vi "MainCamera.vi"() -> ()   [LabVIEW 2018]
uses:
  VisionLibrariesXimea/xiLib/xiLIB_64bit/xiLIB/xiCamLib/xiLIB/Typedefs/xiLIB - PRM_Type.ctl
  VisionLibrariesXimea/xiLib/xiLIB_64bit/xiLIB/xiCamLib/xiLIB/Typedefs/xiLIB - PRM_Function.ctl
  VisionLibrariesXimea/xiLib/xiLIB_64bit/xiLIB/xiCamLib/xiCam/PRM/IMG_FORMAT/IMG_DATA_FORMAT.ctl
  VisionLibrariesXimea/xiLib/xiLIB_64bit/xiLIB/xiCamLib/xiCam/PRM/PRM/PRM_v2.ctl
  <vilib>/Utility/miscctls.llb/LVPointDoubleTypeDef.ctl
  typedef/StateMachineControl.ctl
  NetworkStream/NetworkStreamReceiverState.ctl
  typedef/StateProcessingLoop.ctl
  typedef/ImageUnit.ctl
  VisionLibrariesXimea/xiLib/xiLIB_64bit/xiLIB/xiCamLib/xiCam/PRM/BUFF_POLICY/BUFF_POLICY.ctl
  typedef/AcquisitionFrame.ctl
  NetworkStream/NetworkStreamData.ctl
  VisionLibrariesXimea/xiLib/xiLIB_64bit/xiLIB/xiCamLib/xiCam/PRM/ACQ_TIMING_MODE/ACQ_TIMING_MODE.ctl
  C:/XIMEA/API/x64/xiApi.NETX64.dll
  References.vi
  VisionLibrariesXimea/xiLib/xiLIB_64bit/xiLIB/xiCamLib/xiLIB/xiLIB - GetPRM_INFO.vi
  VisionLibrariesXimea/xiLib/xiLIB_64bit/xiLIB/xiCamLib/xiCam/Methods/xiCam - GetParam_Float.vi
  VisionLibrariesXimea/xiLib/xiLIB_64bit/xiLIB/xiCamLib/xiCam/Methods/xiCam - GetParam_String.vi
  Read and Save Files/FileType.ctl
  General Libraries/myFFT.lvlib
  Read and Save Files/RW_Protocols.lvlib
  General Libraries/Photon Filtering.lvlib
  General Libraries/statistics.lvlib
  NetworkStream/NetworkStream.lvlib
  <vilib>/dex/Stream Element Allocation Mode.ctl
  NetworkStream/NetworkStreamStateMachineVariable.ctl
  Shared program Control/MasterStatus.ctl
  Shared program Control/MySharedVariables.lvlib
panel:
  out "command error":errorcluster
  out "error out":errorcluster
  in  "?":T1(tab)
  in  "Stop Button":bool
  in  "Play Button":bool
  out "current sequence count":i32=10 min=1
  in  "Total sframe":i32=10 min=1
  in  "play sequence":bool
  in  "running mode":T2=enum."free run"
  out "status analysis":T2
  in  "buffer frames":i64=300
  out "# elements queue":i32
  in  "data analysis on":bool=TRUE
  out "efficiency to Main":dbl
  in  "data packing":bool
  in  "recent frame":bool
  in  "software Trigger":bool
  in  "Trigger ON":bool
  in  "Exposure (us)":i32(slide)=10 caption="Exposure (us) 1us - 1s steps of 1us" min=1 max=1000000 scale=0.9..5000.0
  in  "Gain":i32(slide) scale=0.0..10.0
  in  "IMG_FORMAT":T3
  in  "FrameRate":dbl(slide)=100.0 min=0.1 max=400.0 scale=0.0..400.0
  in  "TIMING MODE":i32
  in  "BUFF_POLICY":T4
  in  "auto-save ?":bool
  in  "name":string="Nbz0Nbx1_"
  in  "input PRM":T5=enum."IMAGE_DATA_FORMAT_RGB32_ALPHA"
  out "Type":T6
  out "Method":T7
  out "output":variant
  in  "is value??":bool
  in  "?":T8(tab)
  in  "Width Y":i32=1024 min=32 max=3424 step=32
  in  "Y-offset":i16=1312 min=0 max=3422 step=32
  in  "update ROI":bool
  out "ROI only":bool
  out "max RAM size (frame)":dbl
  in  "infos":bool
  in  "Save As Button":bool
  out "no frame dropping":bool
  out "Intensity Graph":u16[][](graph)
  in  "subwindow control":T10={"2^n : x"=10, "2^n : y"=10, "lower left box Position"={"X"=0.0, "Y"=0.0}, "Height (def 3424)"=0, "Width (def 4704)"=0} {"Width (def 4704)" min=32 max=3264; "Height (def 3424)" min=2 max=2634; "2^n : y" min=1 max=13; "2^n : x" min=1 max=13}
  out "time for acquire":dbl[unit] format="%#_2p"
  out "Enum":T11
  out "Network Stream State Indicator":T12
  out "skipped frames infos":T13
  out "loop":dbl[unit]
  out "required (Bytes) for single image":i32
  out "RAM size (frame)":dbl
  in  "Width X":i32=1024 min=32 max=4704 step=32
  in  "X-offset":i32=1760 min=0 max=2048 step=32
  out "buffer queue size":i32
  out "unit":string
  in  "minus BG":bool
  out "Ptot":dbl format="%#_4p"
  out "% saturation":dbl
  out "FFT":dbl[][](graph)
  in  "FFT int/phase":bool=TRUE
  in  "Filter on/off":bool=TRUE
  in  "filtered int/phase":bool=TRUE
  in  "Mask ON":bool
  out "filtered  FFT":dbl[][](graph)
  in  "unit":T14
  in  "Pause log":bool
  in  "info for log saving":string
  in  "clear graph":bool
  out "Waveform Chart":dbl(graph)
  out "timestamp":dbl
  out "shot noise std":dbl
  out "n":i32=10 min=1
  out "std":dbl
  out "mu":dbl
  out "STD":dbl[][](graph)
  out "MU":dbl[][](graph)
  in  "start stats":bool
  in  "Naverage 2D":i32=10
  in  "save name":string="phase"
  in  "start network scan":bool
  out "std scan":dbl
  out "mean scan":dbl
  out "network scan":dbl(graph)
  out "Sequence Number":u64
  in  "view snaps":bool
  in  "default BG":bool
  in  "Tab Control":T15(tab)
  out "BG":dbl[][](graph)
  in  "Snap":bool
  in  "Snap 2":bool
  out "REF":dbl[][](graph)
  in  "Snap 3":bool
  out "MAIN":dbl[][](graph)
  in  "Snap 4":bool
  out "REF+MAIN":dbl[][](graph)
  in  "phi(2) X":dbl
  in  "phi(2) Z":dbl
  in  "phi(1) X":dbl
  in  "phi(1) Z":dbl
  in  "Target Folder 2":path
  out "reconstructed image":dbl[][](graph)
  out "FFT acquire Graph":dbl[][](graph)
  in  "sequence list":i32[](listbox)
  in  "update loop":bool
  in  "N average":i32=3 min=1
  out "time for acquire":dbl[unit]
  out "timeout":bool=TRUE
  in  "Save result":bool
  in  "name 2":string="myResult"
  out "fft cluster":T16
  in  "sequence NbX NbZ":dbl[][](array[numeric])
  in  "fft cluster acquisition":T16
  in  "result array":dbl[][](array[numeric])
  out "sequence cluster":T17
  out "Array":i32[](array[numeric])
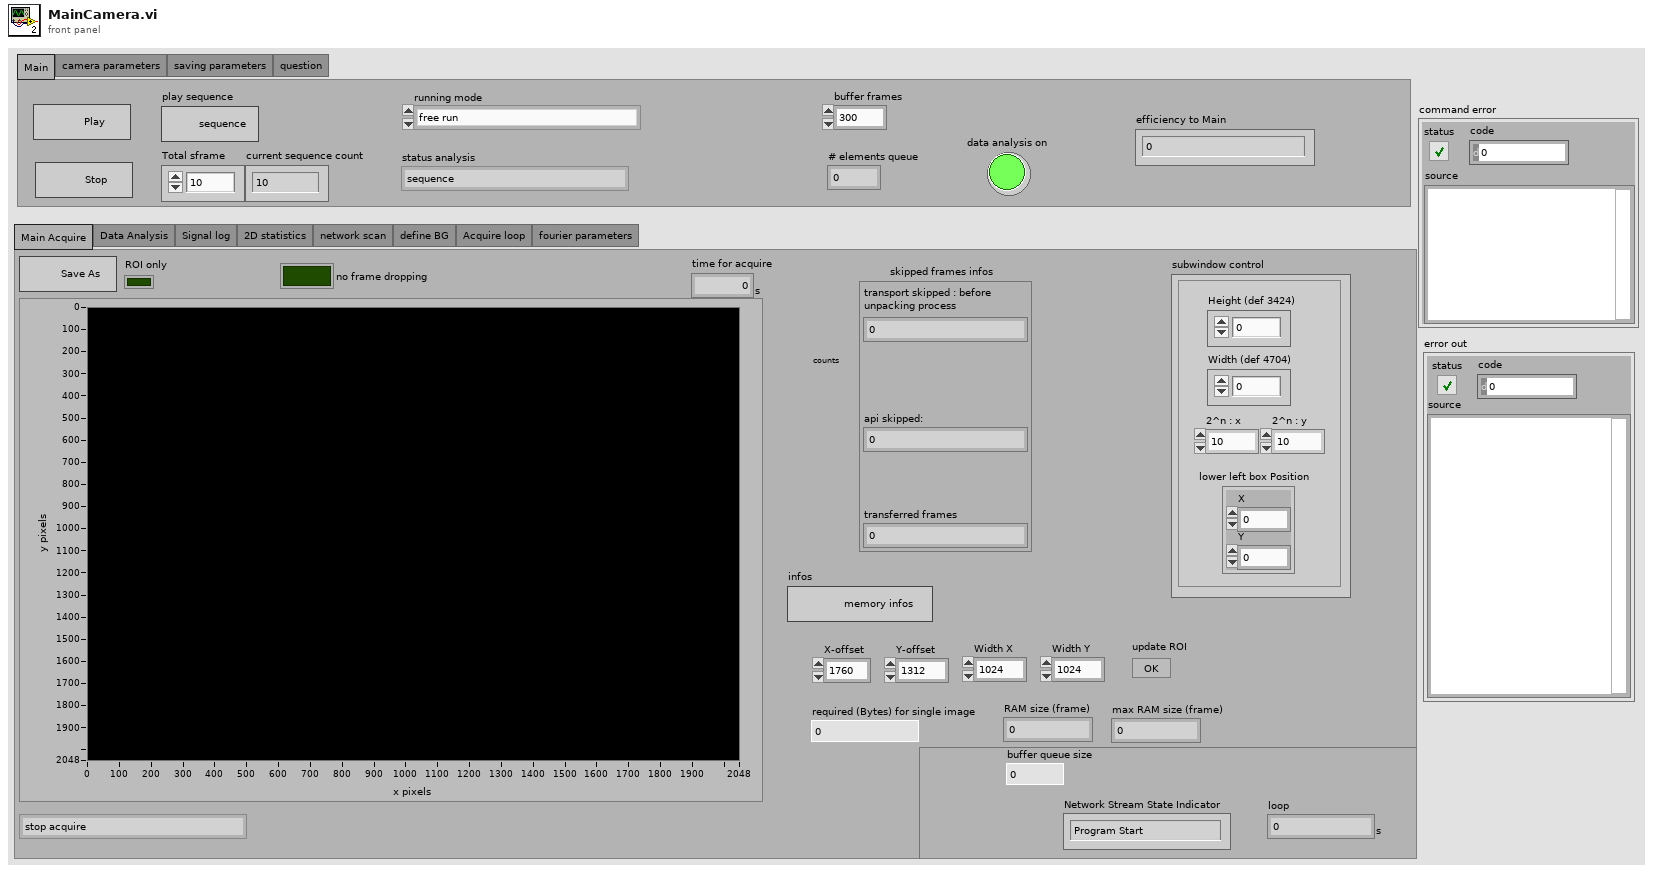
[diagram p1: front panel]
types:
  T1 = enum32{"Main", "camera parameters", "saving parameters", "question"}
  T2 = typedef "StateProcessingLoop.ctl" = enum16{"sequence", "Snap REF+MAIN", "Snap MAIN", "Snap REF", "Snap BG", "network sequence", "free run", "statistics"}
  T3 = typedef "IMG_DATA_FORMAT.ctl" = enum16{"MONO8", "MONO16", "RGB24", "RGB32", "RGBPLANAR", "RAW8", "RAW16"}
  T4 = typedef "BUFF_POLICY.ctl" = enum16{"UNSAFE", "SAFE"}
  T5 = typedef "PRM_v2.ctl" = enum16{"ACQ_BUFFER_SIZE", "ACQ_FRAME_BURST_COUNT", "ACQ_TIMING_MODE", "ACQ_TRANSPORT_BUFFER_SIZE", "AE_MAX_LIMIT", "AEAG", "AEAG_LEVEL", "API_VERSION", "AG_MAX_LIMIT", "APPLY_CMS", "AUTO_BANDWIDTH_CALCULATION", "AUTO_WB", "AVAILABLE_BANDWIDTH", "AVAILABLE_BANDWIDTH_MAX", "AVAILABLE_BANDWIDTH_MIN", "BPC", "BUFFER_POLICY", "BUFFERS_QUEUE_SIZE", "CC_MATRIX_00", "CC_MATRIX_01", "CC_MATRIX_02", "CC_MATRIX_03", "CC_MATRIX_10", "CC_MATRIX_11", "CC_MATRIX_12", "CC_MATRIX_13", "CC_MATRIX_20", "CC_MATRIX_21", "CC_MATRIX_22", "CC_MATRIX_23", "CC_MATRIX_30", "CC_MATRIX_31", "CC_MATRIX_32", "CC_MATRIX_33", "CHIP_TEMP", "CMS", "COLOR_FILTER_ARRAY", "COOLING", "DEBOUNCE_EN", "DEBOUNCE_POL", "DEBOUNCE_T0", "DEBOUNCE_T1", "DEBUG_LEVEL", "DEFAULT_CC_MATRIX", "DEVICE_INSTANCE_PATH", "DEVICE_MODEL_ID", "DEVICE_NAME", "DEVICE_SN", "DEVICE_TYPE", "DEVICE_USER_ID", "DOWNSAMPLING", "DOWNSAMPLING_MAX", "DOWNSAMPLING_MIN", "DOWNSAMPLING_TYPE", "DRV_VERSION", "EXP_PRIORITY", "EXPOSURE", "EXPOSURE_DIRECT_UPDATE", "EXPOSURE_MAX", "EXPOSURE_MIN", "FFS_FILE_NAME", "FPGA1_VERSION", "FRAMERATE", "FRAMERATE_MAX", "FRAMERATE_MIN", "FREE_FFS_SIZE", "GAIN", "GAIN_DIRECT_UPDATE", "GAIN_MAX", "GAIN_MIN", "GAMMAC", "GAMMAY", "GPI_LEVEL", "GPI_MODE", "GPI_SELECTOR", "GPI_SELECTOR_MAX", "GPI_SELECTOR_MIN", "GPO_MODE", "GPO_SELECTOR", "GPO_SELECTOR_MAX", "GPO_SELECTOR_MIN", "HDR", "HDR_T1", "HDR_T2", "HEIGHT", "HEIGHT_MAX", "HEIGHT_MIN", "HOUSE_TEMP", "IMAGE_DATA_FORMAT", "IMAGE_IS_COLOR", "INPUT_CMS_PROFILE", "IS_COOLED", "IS_DEVICE_EXIST", "KNEEPOINT1", "KNEEPOINT2", "LED_MODE", "LED_SELECTOR", "LED_SELECTOR_MAX", "LED_SELECTOR_MIN", "LIMIT_BANDWIDTH", "LIMIT_BANDWIDTH_MAX", "LIMIT_BANDWIDTH_MIN", "LUT_EN", "LUT_INDEX", "LUT_INDEX_MAX", "LUT_INDEX_MIN", "LUT_VALUE", "LUT_VALUE_MAX", "LUT_VALUE_MIN", "MANUAL_WB", "MCU1_VERSION", "MCU2_VERSION", "OFFSET_X", "OFFSET_X_MAX", "OFFSET_X_MIN", "OFFSET_Y", "OFFSET_Y_MAX", "OFFSET_Y_MIN", "OUTPUT_CMS_PROFILE", "OUTPUT_DATA_BIT_DEPTH", "OUTPUT_DATA_PACKING", "READ_FILE_FFS", "RECENT_FRAME", "SENSOR_DATA_BIT_DEPTH", "SENSOR_MODE", "SENSOR_TAPS", "SHARPNESS", "SHUTTER_TYPE", "TARGET_TEMP", "TRG_DELAY", "TRG_SELECTOR", "TRG_SOFTWARE", "TRG_SOURCE", "USED_FFS_SIZE", "WB_KB", "WB_KG", "WB_KR", "WIDTH", "WIDTH_MAX", "WIDTH_MIN", "WRITE_FILE_FFS", "ACQ_BUFFER_SIZE_UNIT", "ACQ_TRANSPORT_BUFFER_COMMIT", "AEAG_ROI_HEIGHT", "AEAG_ROI_OFFSET_X", "AEAG_ROU_OFFSET_Y", "AEAG_ROI_WIDTH", "API_CONTEXT_LIST", "BINNING_HORIZONTAL", "BINNING_SELECTOR", "BINNING_VERTICAL", "COLUMN_FPN_CORRECTION", "COUNTER_SELECTOR", "COUNTER_VALUE", "DECIMATION_HORIZONTAL", "DECIMATION_SELECTOR", "DECIMATION_VERTICAL", "DEVICE_ID", "DEVICE_LOCATION_PATH", "DEVICE_MANIFEST", "DEVICE_RESET", "DEVICE_SENS_SN", "EXPOSURE_BURST_COUNT", "FFS_ACCESS_KEY", "GAIN_SELECTOR", "HW_REVISION", "IMAGE_BLACK_LEVEL", "IMAGE_DATA_BIT_DEPTH", "IMAGE_DATA_FORMAT_RGB32_ALPHA", "IMAGE_PAYLOAD_SIZE", "LENS_APERTURE_VALUE", "LENS_FEATURE", "LENS_FEATURE_SELECTOR", "LENS_FOCAL_LENGTH", "LENS_FOCUS_DISTANCE", "LENS_FOCUS_MOVE", "LENS_FOCUS_MOVEMENT_VALUE", "LENS_MODE", "OUTPUT_DATA_PACKING_TYPE", "SENSOR_CLOCK_FREQ_HZ", "SENSOR_CLOCK_FREQ_INDEX", "SENSOR_FEATURE_SELECTOR", "SENSOR_FEATURE_VALUE", "SENSOR_OUTPUT_CHANNEL_COUNT", "TRANSPORT_PIXEL_FORMAT", "TS_RST_MODE", "TS_RST_SOURCE"}
  T6 = typedef "xiLIB - PRM_Type.ctl" = enum16{"Int32", "Float", "String", "DOWNSAMPLING_TYPE", "IMAGE_DATA_FORMAT", "BUFFER_POLICY", "TRG_SOURCE", "GPI", "GPO", "ACQ_TIMING_MODE", "BINNING_PATTERN", "BINNING_SELECTOR", "CMS_MODE", "COUNTER_SELECTOR", "DEBUG_LEVEL", "DECIMATION_PATTERN", "DECIMATION_SELECTOR", "GAIN_SELECTOR_TYPE", "LED_MODE", "LENS_FEATURE_SELECTOR", "LENS_MODE", "OUTPUT_DATA_PACKING_TYPE", "SENSOR_FEATURE_SELECTOR", "SHUTTER_TYPE", "TRG_SELECTOR", "TS_RST_MODE", "TS_RST_SOURCE"}
  T7 = typedef "xiLIB - PRM_Function.ctl" = enum16{"Get / Set", "Get", "Set"}
  T8 = enum32{"Main Acquire", "Data Analysis", "Signal log", "2D statistics", "network scan", "define BG", "Acquire loop", "fourier parameters"}
  T9 = typedef "LVPointDoubleTypeDef.ctl" = cluster{"X":dbl, "Y":dbl}
  T10 = cluster{"2^n : x":i8, "2^n : y":i8, "lower left box Position":T9, "Height (def 3424)":i32, "Width (def 4704)":i32}
  T11 = typedef "StateMachineControl.ctl" = enum16{"stop acquire", "acquire sequence", "wait", "start acquire sequence", "start acquire", "acquire"}
  T12 = typedef "NetworkStream.lvlib/NetworkStreamReceiverState.ctl" = enum16{"Program Start", "Waiting for connection", "Connected", "Connection lost", "Exit", "Unhandled Exception"}
  T13 = cluster{"transport skipped : before \nunpacking process ":i32, "api skipped: ":i32, "transferred frames":i32}
  T14 = typedef "ImageUnit.ctl" = enum16{"Nphotons", "Efficiency", "I(uW/cm^2)", "I(nW/cm^2)", "Nelectrons", "I[W/cm^2]", "counts"}
  T15 = enum32{"No field", "Ref only", "Main only", "Main + Ref no US"}
  T16 = cluster{"dFx":dbl, "dFy":dbl, "Nx":i32, "Ny":i32, "FxMax":dbl, "FyMax":dbl, "Xwidth":dbl, "Ywidth":dbl, "dx":dbl, "dy":dbl, "Fx points":dbl[], "X points":dbl[], "Y points":dbl[], "Fy points":dbl[]}
  T17 = cluster{"TypeOfSequence":string, "FreqSonde":dbl, "NbHemicycle":dbl, "Tau_cam":dbl, "DurWaveform":dbl, "Prof":dbl, "Nevent":i32, "nuX0":dbl, "nuZ0":dbl}
  T18 = typedef "NetworkStream.lvlib/NetworkStreamData.ctl" = cluster{"Command/Status":string, "Data":variant, "Session Hash":u64, "Sequence Number":u64}
  T19 = typedef "AcquisitionFrame.ctl" = cluster{"data array":u8[], "nframe":i32, "sframe":i32, "nframe0":i32, "data format":i32, "is sequence running ?":bool, "timestamp":dbl}
  T20 = typedef "ACQ_TIMING_MODE.ctl" = enum16{"FREE_RUN", "FRAME_RATE"}
  T21 = typedef "NetworkStream.lvlib/NetworkStreamStateMachineVariable.ctl" = cluster{"Network Stream Reader Endpoint":refnum<k21>, "Last Received Sequence Number":u64}
  T22 = typedef "Stream Element Allocation Mode.ctl" = u32
  T23 = cluster{"MU(1)":dbl[][], "MU(2)":dbl[][], "Ptot(1)":dbl, "Ptot(2)":dbl, "n":i32}
  T24 = cluster{"transport skipped":i32, "api skipped":i32, "transfert skipped":i32}
  T25 = typedef "MySharedVariables.lvlib/MasterStatus.ctl" = cluster{"Camera done":bool, "Tektronik done":bool, "Motors done":bool, "Gage done":bool}[]
  T26 = typedef "RW_Protocols.lvlib/FileType.ctl" = enum16{"png", "csv", "tiff", "dat", "bin", "txt"}
  T27 = cluster{"Filter on/off":bool, "filtered int/phase":bool, "Mask ON":bool, "FFT int/phase":bool}
  T28 = typedef "Photon Filtering.lvlib/OutputPhotonCluster.ctl" = cluster{"Unfiltered":dbl[][], "Ifft":dbl[][], "Ptot":dbl, "Tagged Photons":dbl[][], "% saturation":dbl, "efficiency":dbl, "variance coeff":dbl}
  T29 = cluster{"Camera done":bool, "Tektronik done":bool, "Motors done":bool, "Gage done":bool}
  T30 = cluster{"phi(1) X":dbl, "phi(1) Z":dbl, "phi(2) X":dbl, "phi(2) Z":dbl}
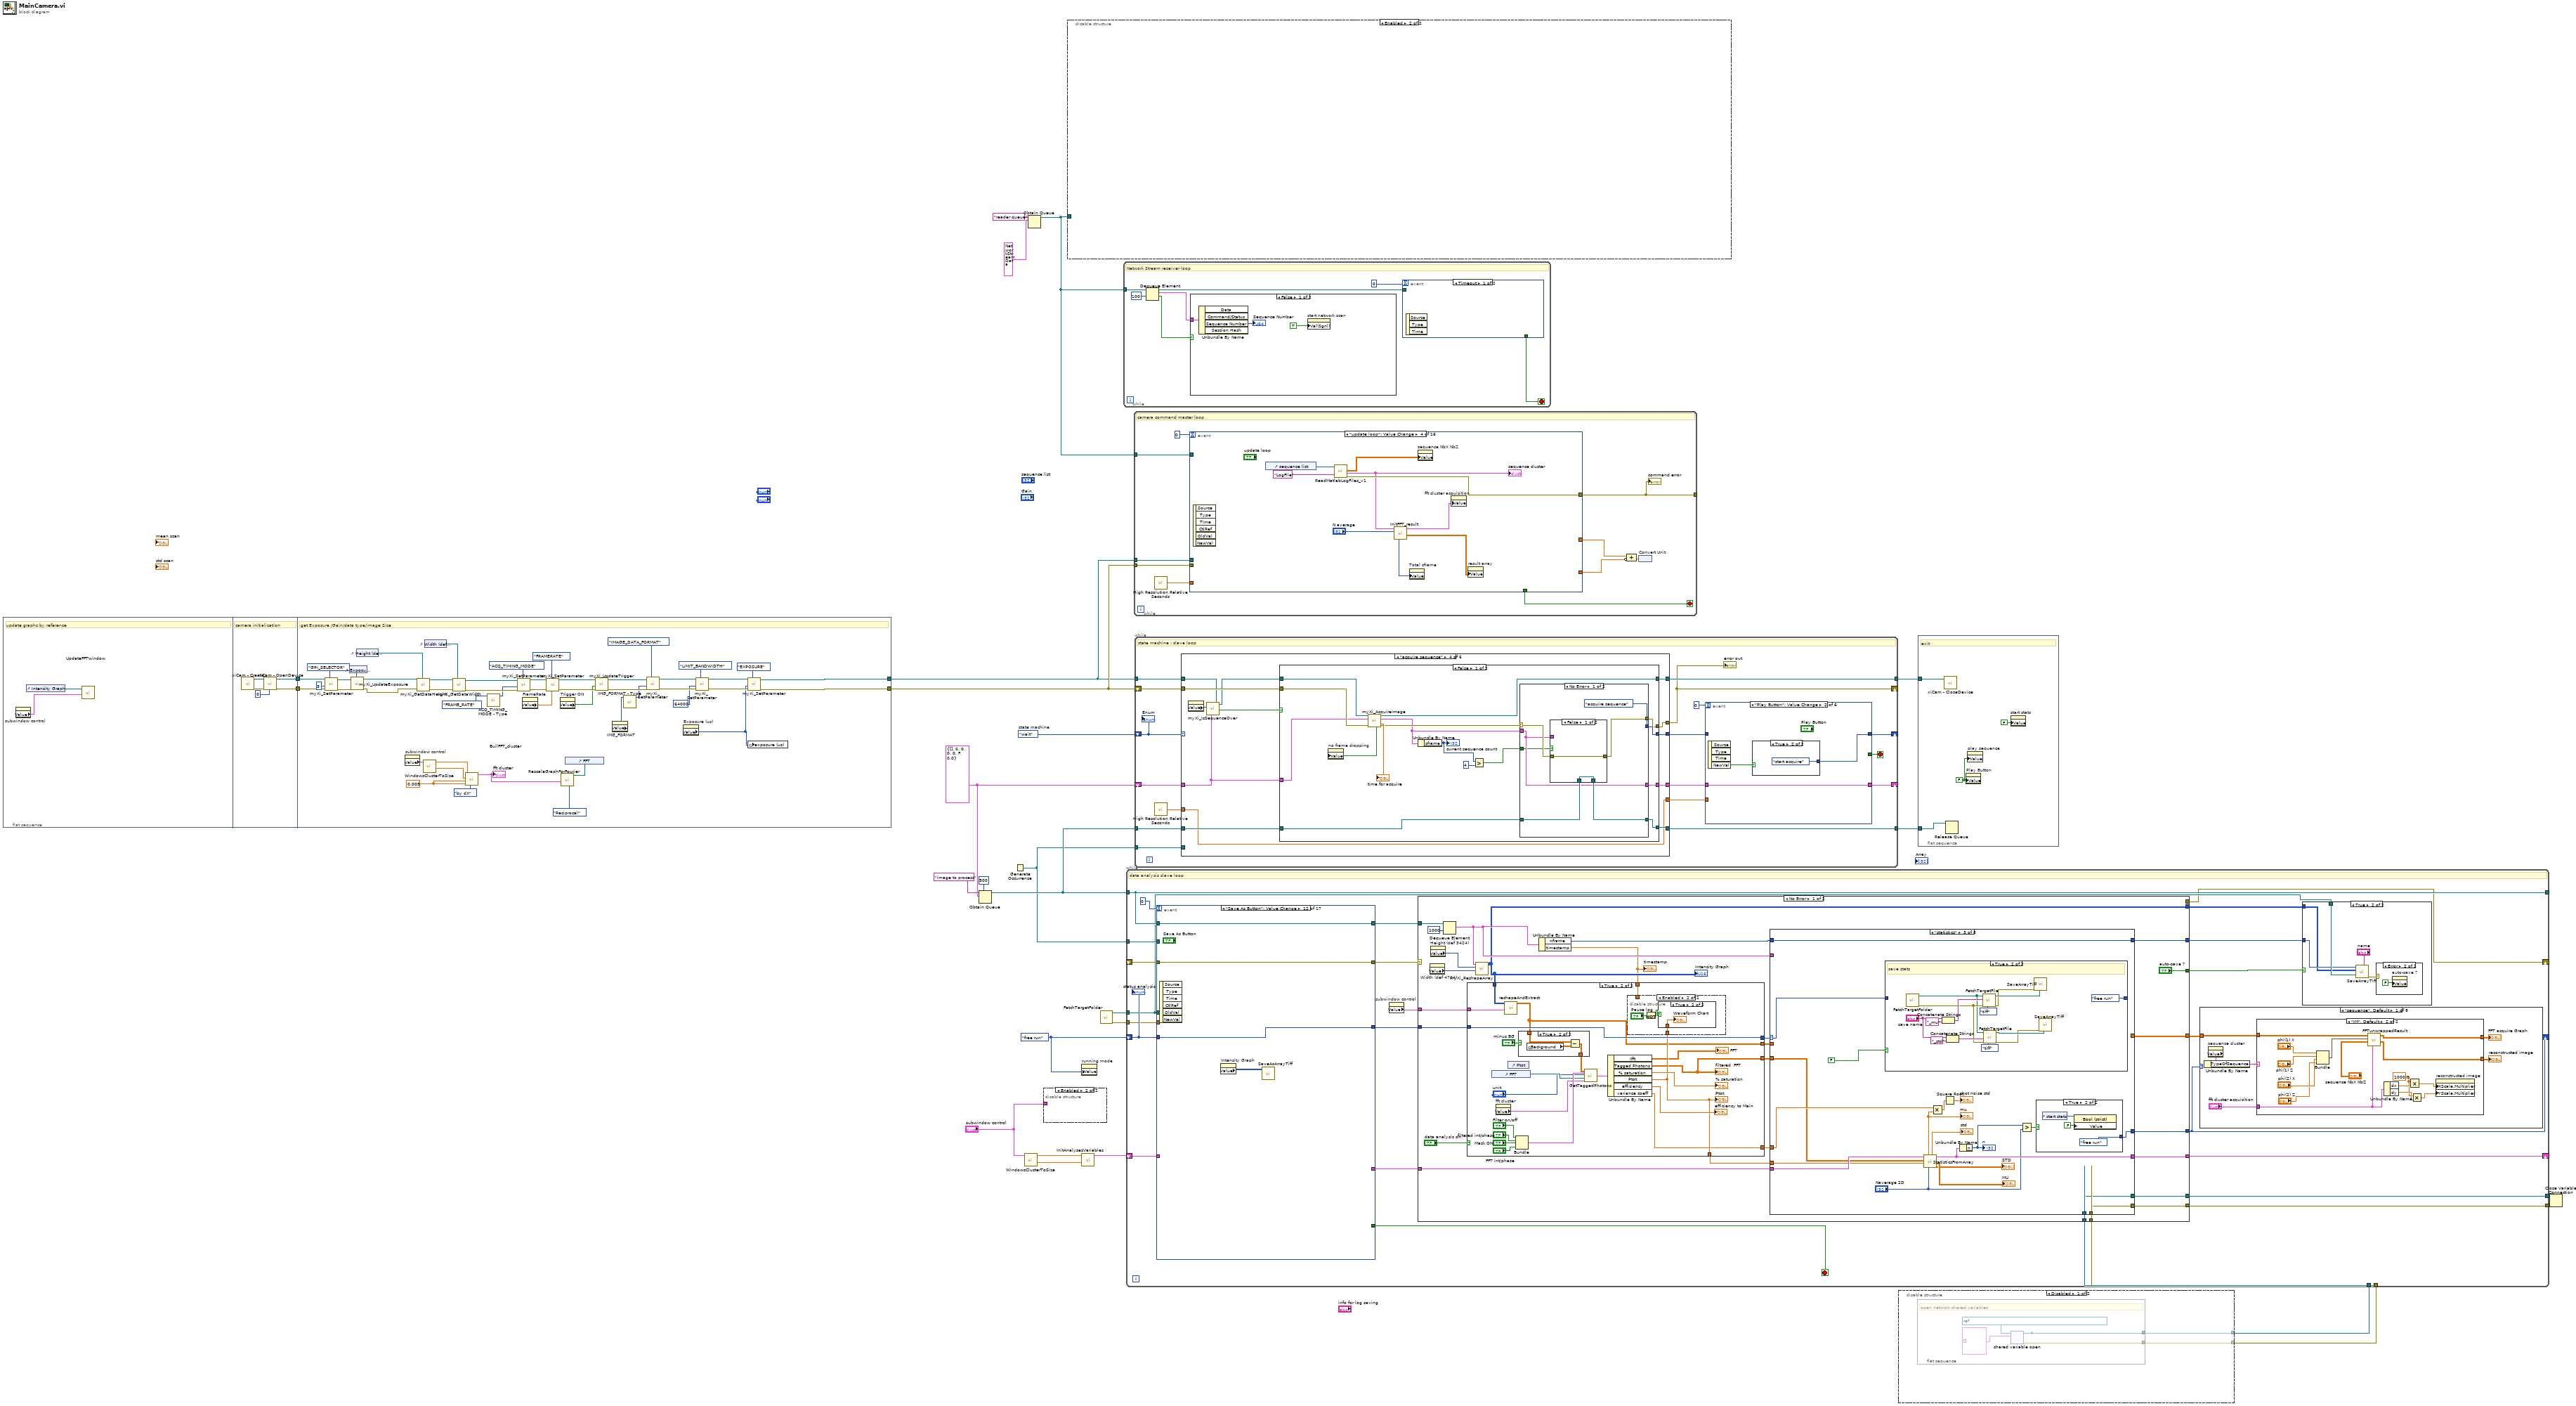
[diagram p0: block diagram]
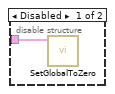
[diagram p2: hidden frame]
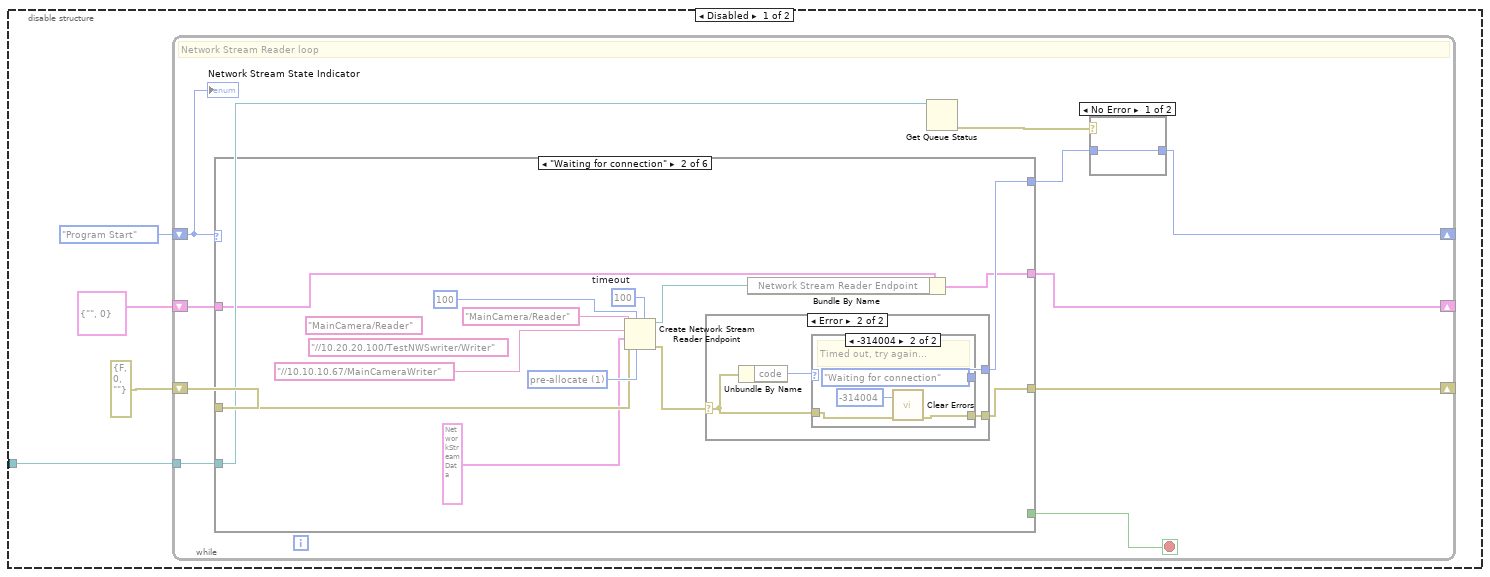
[diagram p4: hidden frame]
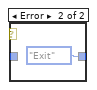
[diagram p5: hidden frame]
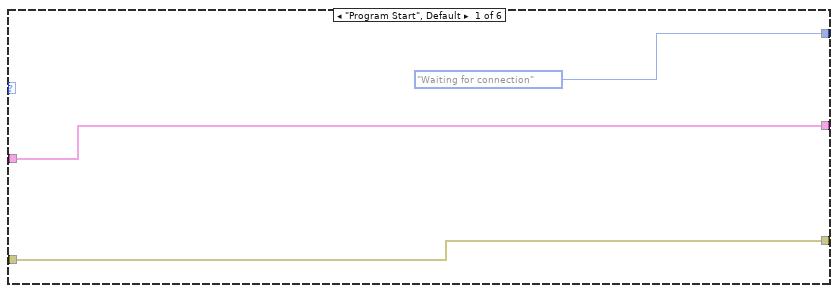
[diagram p6: hidden frame]
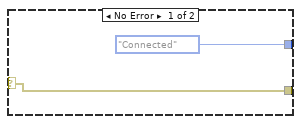
[diagram p7: hidden frame]
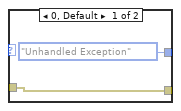
[diagram p8: hidden frame]
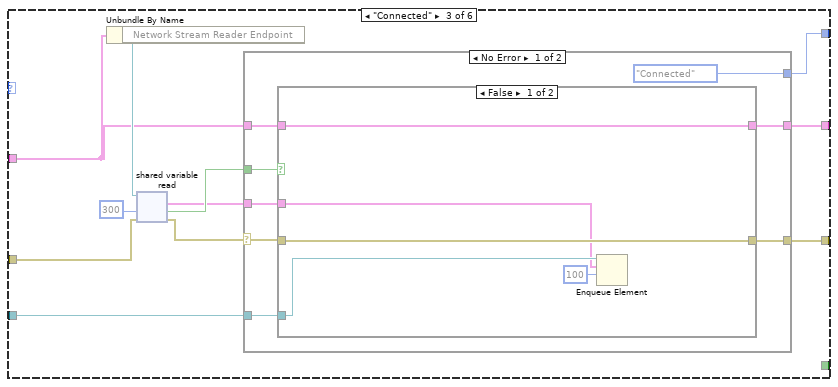
[diagram p9: hidden frame]
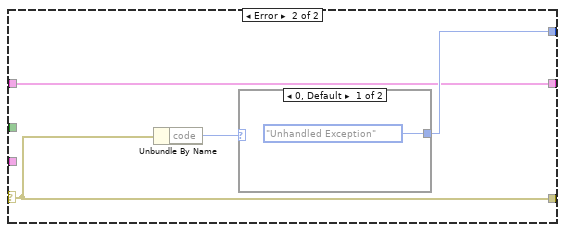
[diagram p11: hidden frame]
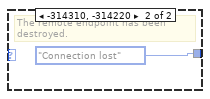
[diagram p12: hidden frame]
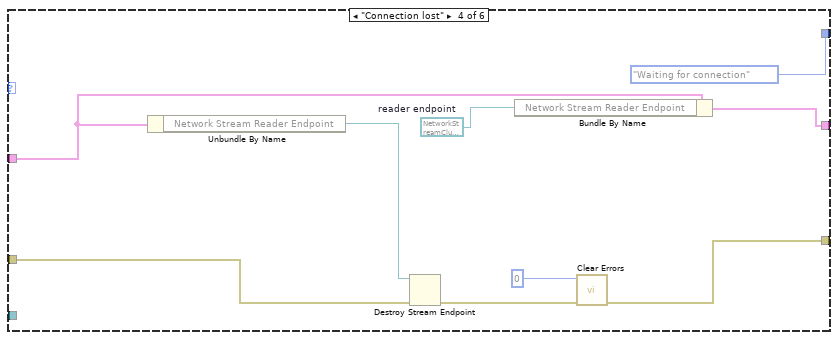
[diagram p13: hidden frame]
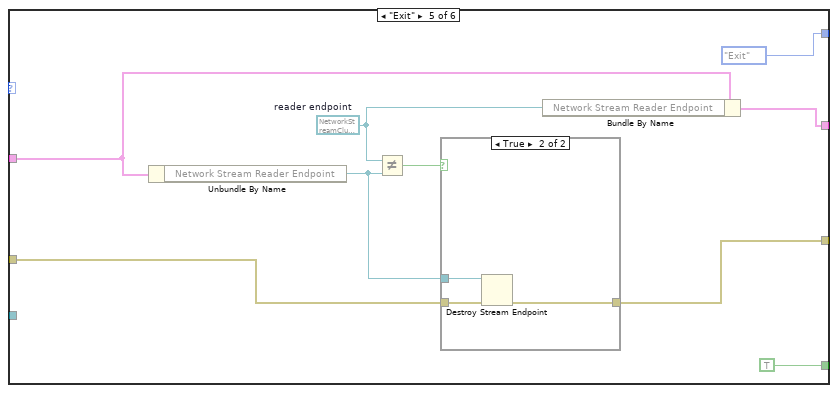
[diagram p14: hidden frame]
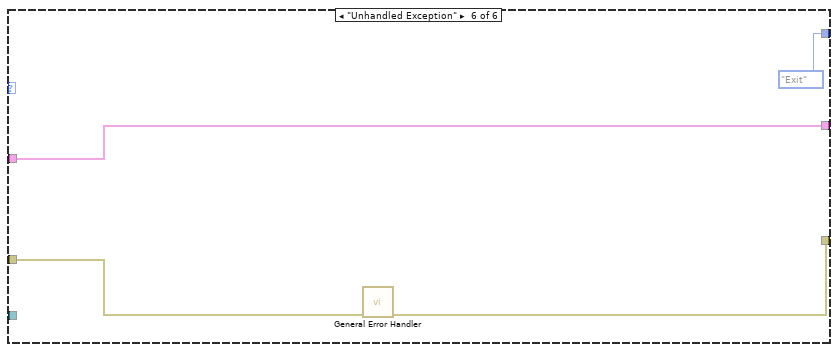
[diagram p16: hidden frame]
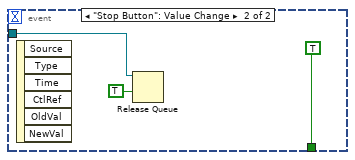
[diagram p18: hidden frame]
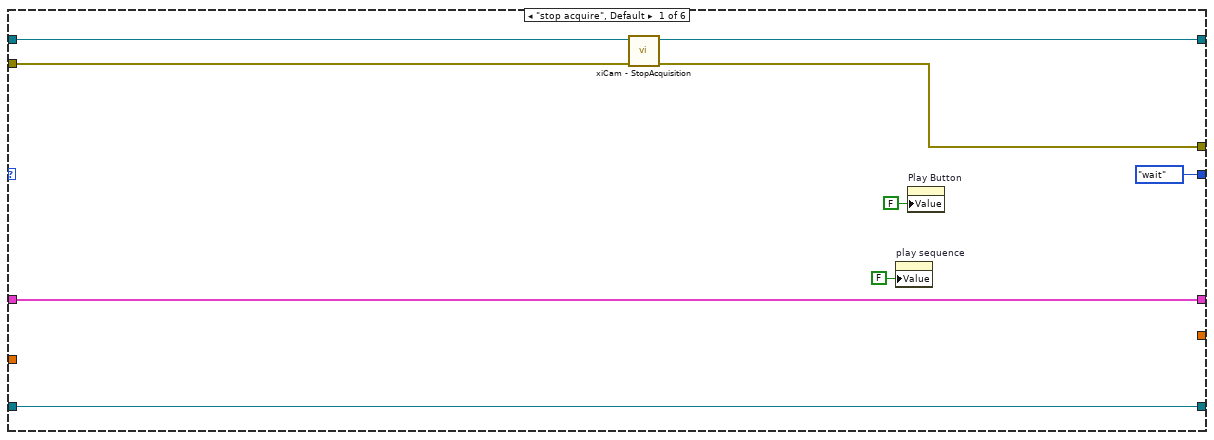
[diagram p19: hidden frame]
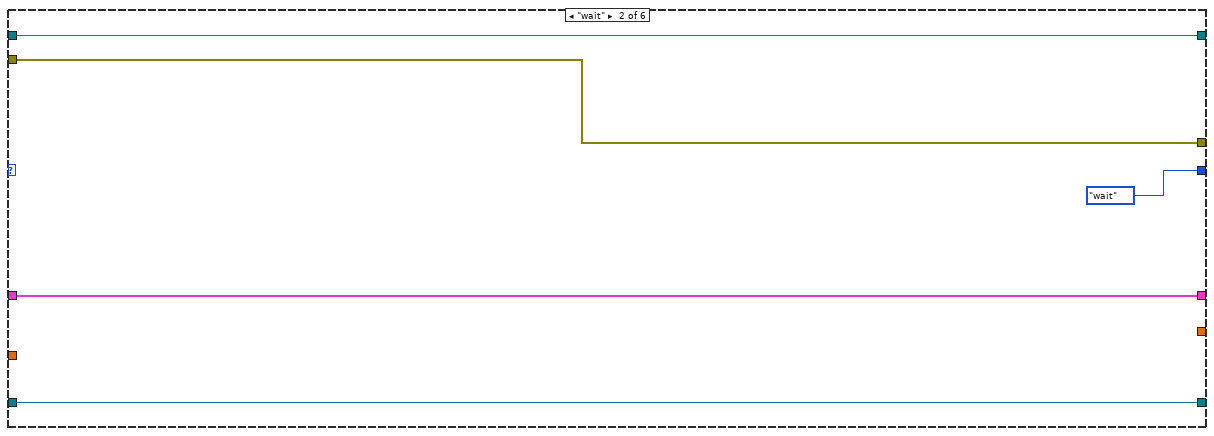
[diagram p20: hidden frame]
diagram:
  w16 = T19 {"data array"=[], "nframe"=0, "sframe"=0, "nframe0"=0, "data format"=0, "is sequence running ?"=FALSE, "timestamp"=0.0} ("acquisition frame")
  w5 = StateProcessingLoop."free run" ("Enum")
  w21 = StateMachineControl."wait"  # state machine
  n1 = flat-sequence {
    tunnel: [w33] -> w24
    tunnel: [w32] -> w23
    tunnel: [w36] -> w26
    tunnel: [w37] -> w22
    tunnel: w24 -> [w72]
    tunnel: w23 -> [w74]
    frame #0 {
      # "update graphs by reference"
      n2 = property on="subwindow control" class="Clust (strict)"() -> ("Value"=w27:T10)  [unwired: 2 in, 2 out]
      n3 = control-ref of="Intensity Graph"() -> (w28:refnum<vi>)
      n4 = call "UpdateFFTwindow.vi"("subwindow IN"=w27, "Intensity Graph"=w28) -> ()  [unwired: 9 in, 1 out]
    }
    frame #1 {
      # "camera initialization"
      n5 = call "xiCam - Create.vi"() -> ("error out"=w30:errorcluster, "new xiCam"=w31:refnum<k24>)  [unwired: 10 in]
      n6 = call "xiCam - OpenDevice.vi"("DevID"=0, "error in (no error)"=w30, "xiCam In"=w31) -> ("error out"=w32:errorcluster, "xiCam Out"=w33:refnum<k24>)  [unwired: 7 in]
    }
    frame #2 {
      w76 = 0.005 ("input X")
      # "get Exposure /Gain/data type/image Size"
      n7 = call "myXi_SetParameter.vi"("input PRM"=PRM_v2."GPI_SELECTOR", "error in"=w74, "input value I32"=3, "xiCam IN"=w72) -> ("error out"=w73:errorcluster, "xiCam Out"=w71:refnum<k24>)  [unwired: 6 in]
      n8 = control-ref of="Exposure (us)"() -> (w81:refnum<vi>)
      n9 = call "myXi_UpdateExposure.vi"("Exposure (us)"=w81, "error in"=w73, "xiCam In"=w71) -> ("error out"=w34:errorcluster, "xiCam Out"=w35:refnum<k24>)  [unwired: 7 in]
      n10 = control-ref of="Height (def 3424)"() -> (w80:refnum<vi>)
      n11 = property on="subwindow control" class="Clust (strict)"() -> ("Value"=w46:T10)  [unwired: 2 in, 2 out]
      n12 = call "myXi_GetDataHeight.vi"("Height"=w80, "error in"=w34, "xiCam In"=w35) -> ("error out"=w78:errorcluster, "xiCam Out"=w79:refnum<k24>)  [unwired: 6 in, 1 out]
      n13 = call "WindowsClusterToSize.vi"("subwindow control 2"=w46) -> ("Ny"=w48:dbl, "Nx"=w47:dbl)  [unwired: 9 in]
      n14 = control-ref of="Width (def 4704)"() -> (w77:refnum<vi>)
      n15 = call "myXi_GetDataWidth.vi"("width"=w77, "error in"=w78, "xiCam In"=w79) -> ("error out"=w64:errorcluster, "xiCam Out"=w65:refnum<k24>)  [unwired: 6 in, 1 out]
      n16 = call "BuilFFT_cluster.vi"("Enum"=enum16{"by dF", "by dX"}."by dX", "input Y"=w76, "input X"=w76, "Ny"=w48, "Nx"=w47) -> ("fft cluster"=w66:T16)  [unwired: 6 in]
      "fft cluster" <- w66
      n17 = call "ACQ_TIMING_MODE - Type.vi"("ACQ TIMING MODE"=ACQ_TIMING_MODE."FRAME_RATE") -> ("ACQ_TIMING_MODE_VALUE"=w61:i32)  [unwired: 9 in, 1 out]
      n18 = call "myXi_SetParameter.vi"("input PRM"=PRM_v2."ACQ_TIMING_MODE", "error in"=w64, "input value I32"=w61, "xiCam IN"=w65) -> ("error out"=w60:errorcluster, "xiCam Out"=w59:refnum<k24>)  [unwired: 6 in]
      n19 = property on="FrameRate" class="Slide (strict)"() -> ("Value"=w58:dbl)  [unwired: 2 in, 2 out]
      n20 = call "myXi_SetParameter.vi"("input value DBL"=w58, "input PRM"=PRM_v2."FRAMERATE", "error in"=w60, "xiCam IN"=w59) -> ("error out"=w56:errorcluster, "xiCam Out"=w55:refnum<k24>)  [unwired: 6 in]
      n21 = property on="Trigger ON" class="Bool (strict)"() -> ("Value"=w54:bool)  [unwired: 2 in, 2 out]
      n22 = control-ref of="FFT"() -> (w68:refnum<vi>)
      n23 = call "RescaleGraphForFourier.vi"("fft reference"=w68, "fft cluster"=w66, "Enum"=enum16{"Reciprocal", "Real"}."Reciprocal") -> ()  [unwired: 8 in]
      n24 = call "myXi_UpdateTrigger.vi"("error in (no error)"=w56, "trigger"=w54, "xiCam IN"=w55) -> ("error out"=w53:errorcluster, "xiCam Out"=w52:refnum<k24>)  [unwired: 7 in]
      n25 = property on="IMG_FORMAT" class="Enum (strict)"() -> ("Value"=w49:T3)  [unwired: 2 in, 2 out]
      n26 = call "IMG_FORMAT - Type.vi"("IMG_FORMAT"=w49) -> ("IMG_FORMAT_VALUE"=w50:i32)  [unwired: 9 in, 1 out]
      n27 = call "myXi_SetParameter.vi"("input PRM"=PRM_v2."IMAGE_DATA_FORMAT", "error in"=w53, "input value I32"=w50, "xiCam IN"=w52) -> ("error out"=w45:errorcluster, "xiCam Out"=w44:refnum<k24>)  [unwired: 6 in]
      n28 = property on="Exposure (us)" class="Slide (strict)"() -> ("Value"=w38:i32)  [unwired: 2 in, 2 out]
      n29 = call "myXi_SetParameter.vi"("input PRM"=PRM_v2."LIMIT_BANDWIDTH", "error in"=w45, "input value I32"=i64 64000, "xiCam IN"=w44) -> ("error out"=w41:errorcluster, "xiCam Out"=w40:refnum<k24>)  [unwired: 6 in]
      n30 = call "myXi_SetParameter.vi"("input PRM"=PRM_v2."EXPOSURE", "error in"=w41, "input value I32"=w38, "xiCam IN"=w40) -> ("error out"=w36:errorcluster, "xiCam Out"=w37:refnum<k24>)  [unwired: 6 in]
      n31 = global write "References.vi" "exposure (us)"(w38) -> ()
    }
  }
  n32 = Obtain Queue(max queue size (-1, unlimited)=500, name (unnamed)="image to process", element data type=w16) -> (queue out=w17:refnum<queue>)  [unwired: 2 in, 2 out]
  n33 = Generate Occurrence() -> (w6:refnum<k4>)
  n34 = call "WindowsClusterToSize.vi"("subwindow control 2"="subwindow control") -> ("Ny"=w1:dbl, "Nx"=w2:dbl)  [unwired: 9 in]
  n35 = Obtain Queue(name (unnamed)="reader queue", element data type=T18 {"Command/Status"="", "Data"=variant, "Session Hash"=0, "Sequence Number"=0} ("NetworkStreamCluster")) -> (queue out=w13:refnum<queue>)  [unwired: 3 in, 2 out]
  n36 = disable-structure shown="Enabled" {
    disable-tunnel: "subwindow control" -> [w82 _]
    frame Disabled {
      n37 = call "SetGlobalToZero.vi"("subwindow control"=w82) -> ()  [unwired: 11 in]
    }
    frame Enabled {
    }
  }
  n38 = disable-structure shown="Enabled" {
    disable-tunnel: w13 -> [w83 _]
    frame Disabled {
      n39 = while {
        shift-right: [w94] -> _
        shift-left: T21 {"Network Stream Reader Endpoint"="", "Last Received Sequence Number"=0} ("StateMachineVariable") -> [w96]
        shift-right: [w89] -> _
        shift-left: NetworkStreamReceiverState."Program Start" -> [w95]
        shift-right: [w93] -> _
        shift-left: errorcluster {"status"=FALSE, "code"=0, "source"=""} ("error out") -> [w91]
        tunnel: w83 -> [w87]
        stop <- w92 stop-if-true
        # "Network Stream Reader loop"
        n40 = case shown="\"Waiting for connection\"" w95 {
          tunnel: [NetworkStreamReceiverState."Waiting for connection" w111 w132 NetworkStreamReceiverState."Waiting for connection" NetworkStreamReceiverState."Exit" NetworkStreamReceiverState."Exit"] -> w90
          tunnel: [w100 w110 w133 w163 w176 w184] -> w93
          tunnel: [w99 w109 w130 w159 w169 w181] -> w94
          tunnel: [_ _ _ _ TRUE _] -> w92
          tunnel: w96 -> [w99 w107 w129 w160 w170 w181]
          tunnel: w91 -> [w100 w106 w128 w162 w171 w182]
          tunnel: w87 -> [_ _ w127 _ _ _]
          frame "Program Start", Default {
          }
          frame "Waiting for connection" {
            (unwired) "MainCamera/Reader" ("reader name")
            (unwired) "//10.20.20.100/TestNWSwriter/Writer" ("writer url")
            w108 = T22 1 items=["allocate as needed", "pre-allocate"] ("element allocation mode")
            w114 = 100  # timeout
            n41 = Create Network Stream Reader Endpoint(5:w114, 6:w108, 7:100 ("reader buffer size"), 8:w106, 9:T18 {"Command/Status"="", "Data"=variant, "Session Hash"=0, "Sequence Number"=0} ("NetworkStreamCluster"), 10:"//10.10.10.67/MainCameraWriter" ("writer url"), 11:"MainCamera/Reader" ("reader name")) -> (0:w112:errorcluster, 3:w104:refnum<k21>)
            n42 = case shown="Error" w112 {
              selector: w112 -> [w115 w118]
              tunnel: [NetworkStreamReceiverState."Connected" w120] -> w111
              tunnel: [w115 w117] -> w110
              frame No Error {
              }
              frame Error {
                n43 = Unbundle By Name(w118) -> ("code"=w119:i32)
                n44 = case shown="-314004" w119 {
                  tunnel: [NetworkStreamReceiverState."Unhandled Exception" NetworkStreamReceiverState."Waiting for connection"] -> w120
                  tunnel: w118 -> [w121 w124]
                  tunnel: [w121 w123] -> w117
                  frame 0, Default {
                  }
                  frame -314004 {
                    # "Timed out, try again..."
                    n45 = call <vilib>:"Clear Errors.vi"("error in (no error)"=w124, "specific error code to clear (0: all)"=-314004) -> ("error out"=w123:errorcluster)  [unwired: 4 in, 1 out]
                  }
                }
              }
            }
            n46 = Bundle By Name(cluster=w107, "Network Stream Reader Endpoint"=w104) -> (w109:T21)
          }
          frame "Connected" {
            n47 = Unbundle By Name(w129) -> ("Network Stream Reader Endpoint"=w131:refnum<k21>)
            n48 = shared-variable-read(w131, w128, 300 ("timeout ms (-1)")) -> (w134:errorcluster, w136:bool, w135:T18)  [unwired: 1 out]
            n49 = case shown="No Error" w134 {
              selector: w134 -> [w143 w156]
              tunnel: w136 -> [w145 _]
              tunnel: w135 -> [w144 _]
              tunnel: [w142 w156] -> w133
              tunnel: [NetworkStreamReceiverState."Connected" w154] -> w132
              tunnel: [w140 w153] -> w130
              tunnel: w129 -> [w139 w153]
              tunnel: w127 -> [w138 _]
              frame No Error {
                n50 = case shown="False" w145 {
                  tunnel: [w149 w152] -> w142
                  tunnel: w143 -> [w149 w152]
                  tunnel: w144 -> [w146 _]
                  tunnel: [w150 w151] -> w140
                  tunnel: w139 -> [w150 w151]
                  tunnel: w138 -> [w148 _]
                  frame False {
                    n51 = Enqueue Element(queue=w148, element=w146, timeout in ms (-1)=100) -> ()  [unwired: 1 in, 3 out]
                  }
                  frame True {
                  }
                }
              }
              frame Error {
                n52 = Unbundle By Name(w156) -> ("code"=w155:i32)
                n53 = case shown="0, Default" w155 {
                  tunnel: [NetworkStreamReceiverState."Unhandled Exception" NetworkStreamReceiverState."Connection lost"] -> w154
                  frame 0, Default {
                  }
                  frame -314310, -314220 {
                    # "The remote endpoint has been destroyed."
                  }
                }
              }
            }
          }
          frame "Connection lost" {
            w166 = refnum<k21> refnum  # reader endpoint
            n54 = Unbundle By Name(w160) -> ("Network Stream Reader Endpoint"=w161:refnum<k21>)
            n55 = Destroy Stream Endpoint(8:w162, 11:w161) -> (0:w165:errorcluster)
            n56 = Bundle By Name(cluster=w160, "Network Stream Reader Endpoint"=w166) -> (w159:T21)
            n57 = call <vilib>:"Clear Errors.vi"("error in (no error)"=w165, "specific error code to clear (0: all)"=0) -> ("error out"=w163:errorcluster)  [unwired: 4 in, 1 out]
          }
          frame "Exit" {
            w172 = refnum<k21> refnum  # reader endpoint
            n58 = Unbundle By Name(w170) -> ("Network Stream Reader Endpoint"=w168:refnum<k21>)
            n59 = Not Equal?(x=w172, y=w168) -> (x != y?=w174:bool)
            n60 = case shown="True" w174 {
              tunnel: [w177 w180] -> w176
              tunnel: w171 -> [w177 w179]
              tunnel: w168 -> [_ w178]
              frame False {
              }
              frame True {
                n61 = Destroy Stream Endpoint(8:w179, 11:w178) -> (0:w180:errorcluster)
              }
            }
            n62 = Bundle By Name(cluster=w170, "Network Stream Reader Endpoint"=w172) -> (w169:T21)
          }
          frame "Unhandled Exception" {
            n63 = call <vilib>:"General Error Handler.vi"("error in (no error)"=w182) -> ("error out"=w184:errorcluster)  [unwired: 10 in, 4 out]
          }
        }
        n64 = Get Queue Status(queue=w87) -> (error out=w88:errorcluster)  [unwired: 2 in, 7 out]
        n65 = case shown="No Error" w88 {
          tunnel: w90 -> [w97 _]
          tunnel: [w97 NetworkStreamReceiverState."Exit"] -> w89
          frame No Error {
          }
          frame Error {
          }
        }
        "Network Stream State Indicator" <- w95
      }
    }
    frame Enabled {
    }
  }
  n66 = property on="running mode" class="Enum (strict)"("Value"=w5) -> ()  [unwired: 2 in, 2 out]
  n67 = call "InitAnalysesVariables.vi"("Ny [rows]"=w1, "Nx [cols]"=w2) -> ("Stat Vars"=w4:T23)  [unwired: 9 in]
  n68 = call "FetchTargetFolder.vi"() -> ("error out"=w7:errorcluster, "Full File Path"=w8:path)  [unwired: 10 in]
  n69 = while {
    tunnel: w13 -> [w185]
    stop <- w191 stop-if-true
    # "Network Stream receiver loop"
    n70 = Dequeue Element(queue=w185, timeout in ms (-1)=100) -> (queue out=w187:refnum<queue>, element=w189:T18, timed out?=w186:bool)  [unwired: 1 in, 1 out]
    n71 = case shown="False" w186 {
      tunnel: w189 -> [w194 _]
      frame False {
        n72 = Unbundle By Name(w194) -> ("Sequence Number"=→"Sequence Number":u64)  [unwired: 3 out]
        n73 = property on="start network scan" class="Bool (strict)"("Val(Sgnl)"=TRUE) -> ()  [unwired: 2 in, 2 out]
      }
      frame True {
      }
    }
    n74 = event shown="[0] Timeout" {
      selector: _ -> [_ _]
      dyn-events: _ -> [_ _]
      timeout: 0 -> [_ _]
      tunnel: [_ TRUE] -> w191
      tunnel: w187 -> [_ w196]
      event Timeout {
        n75 = event-data() -> ()  [unwired: 1 in, 3 out]
      }
      event "Stop Button": Value Change {
        n76 = event-data() -> ()  [unwired: 1 in, 6 out]
        n77 = Release Queue(queue=w196, force destroy? (F)=TRUE) -> ()  [unwired: 1 in, 3 out]
      }
    }
  }
  n78 = while {
    tunnel: w22 -> [w206]
    tunnel: w26 -> [w205]
    tunnel: [w204] -> _
    tunnel: w13 -> [w198]
    stop <- w207 stop-if-true
    # "camera command master loop"
    n79 = call <vilib>:"High Resolution Relative Seconds.vi"() -> ("relative seconds"=w199:dbl)
    n80 = event shown="[3] \"update loop\": Value Change" {
      selector: _ -> [_ _ _ _ _ _ _ _ _ _ _ _ _ _ _ _]
      dyn-events: _ -> [_ _ _ _ _ _ _ _ _ _ _ _ _ _ _ _]
      timeout: 0 -> [_ _ _ _ _ _ _ _ _ _ _ _ _ _ _ _]
      tunnel: [_ _ _ _ _ TRUE _ _ _ _ _ _ _ _ _ _] -> w207
      tunnel: w206 -> [w209 w233 _ _ w248 _ w258 w275 w280 w285 w311 w332 w351 _ w357 w363]
      tunnel: w205 -> [w210 w232 _ _ w247 w250 w257 w274 w278 w289 w309 w331 w350 w353 w356 w362]
      tunnel: [w208 w220 _ w242 w246 w250 w252 w268 w279 w292 w308 w330 w349 w353 w355 w359] -> w204
      tunnel: [w213 _ _ _ _ _ _ _ _ _ _ _ _ _ _ _] -> w201
      tunnel: w199 -> [w213 _ _ _ _ _ _ _ _ _ _ _ _ _ _ _]
      tunnel: [w212 _ _ _ _ _ _ _ _ _ _ _ _ _ _ _] -> w200
      tunnel: w198 -> [_ _ _ _ _ _ _ _ _ _ _ _ _ _ _ _]
      event Timeout {
        n81 = event-data() -> ()  [unwired: 1 in, 3 out]
        n82 = flat-sequence {
          tunnel: [w214] -> w211
          tunnel: [w219] -> w212
          tunnel: w211 -> [w219]
          tunnel: w210 -> [w217]
          tunnel: w209 -> [w218]
          tunnel: [w216] -> w208
          frame #0 {
            n83 = call <vilib>:"High Resolution Relative Seconds.vi"() -> ("relative seconds"=w214:dbl)
          }
          frame #1 {
            # "stats on frame rate"
            n84 = call "myXi_GetDataFrameStats.vi"("error in (no error)"=w217, "xiCam IN"=w218) -> ("error out"=w216:errorcluster, "skipped frame"=→"skipped frames infos":T24)  [unwired: 7 in, 1 out]
          }
        }
      }
      event "infos": Value Change {
        n85 = event-data() -> ()  [unwired: 1 in, 6 out]
        n86 = call "xiCam - GetParam_Int32.vi"("PRM"=PRM_v2."IMAGE_PAYLOAD_SIZE", "error in (no error)"=w232, "xiCam In"=w233) -> ("error out"=w230:errorcluster, "xiCam Out"=w231:refnum<k24>, "Int32_Value"=w227:i32)  [unwired: 6 in]
        "required (Bytes) for single image" <- w227
        n87 = call "xiCam - GetParam_Int32.vi"("PRM"=PRM_v2."ACQ_BUFFER_SIZE", "error in (no error)"=w230, "xiCam In"=w231) -> ("error out"=w224:errorcluster, "xiCam Out"=w223:refnum<k24>, "Int32_Value"=w229:i32)  [unwired: 6 in]
        n88 = Divide(x=2147483647, y=w227) -> (x/y=→"max RAM size (frame)":dbl)
        n89 = Divide(x=w229, y=w227) -> (x/y=→"RAM size (frame)":dbl)
        n90 = call "xiCam - GetParam_Int32.vi"("PRM"=PRM_v2."BUFFERS_QUEUE_SIZE", "error in (no error)"=w224, "xiCam In"=w223) -> ("error out"=w220:errorcluster, "Int32_Value"=→"buffer queue size":i32)  [unwired: 6 in, 1 out]
      }
      event "ROI only": Value Change {
        n91 = event-data() -> ()  [unwired: 1 in, 6 out]
      }
      event "update loop": Value Change {
        n92 = event-data() -> ()  [unwired: 1 in, 6 out]
        n93 = control-ref of="sequence list"() -> (w244:refnum<vi>)
        n94 = call "ReadMatlabLogFiles_v1.vi"("FileName"="LogFile", "sequence list REF"=w244) -> ("error out"=w242:errorcluster, "sequence cluster"=w240:T17, "sequence NbX NbZ"=w241:dbl[][])  [unwired: 4 in, 3 out]
        "sequence cluster" <- w240
        n95 = call "InitFFT_result.vi"("N average"="N average", "sequence IN"=w240) -> ("initialized frame array"=w237:dbl[][], "fft cluster"=w236:T16, "Stot"=w238:i32)  [unwired: 6 in, 1 out]
        n96 = property on="Total sframe" class="DigNum (strict)"("Value"=w238) -> ()  [unwired: 2 in, 2 out]
        n97 = property on="sequence NbX NbZ" class="Arr (strict)"("Value"=w241) -> ()  [unwired: 2 in, 2 out]
        n98 = property on="fft cluster acquisition" class="Clust (strict)"("Value"=w236) -> ()  [unwired: 2 in, 2 out]
        n99 = property on="result array" class="Arr (strict)"("Value"=w237) -> ()  [unwired: 2 in, 2 out]
      }
      event "Exposure (us)": Value Change {
        n100 = event-data() -> ("NewVal"=w245:i32)  [unwired: 1 in, 5 out]
        n101 = call "myXi_SetParameter.vi"("input PRM"=PRM_v2."EXPOSURE", "error in"=w247, "input value I32"=w245, "xiCam IN"=w248) -> ("error out"=w246:errorcluster)  [unwired: 6 in, 1 out]
        n102 = global write "References.vi" "exposure (us)"(w245) -> ()
      }
      event "Stop Button": Value Change {
        n103 = event-data() -> ()  [unwired: 1 in, 6 out]
      }
      event "is value??": Value Change {
        n104 = event-data() -> ()  [unwired: 1 in, 6 out]
        n105 = call "myXi_GetParameter.vi"("input PRM"="input PRM", "error in"=w257, "xiCam IN"=w258) -> ("error out"=w252:errorcluster, "Type"=→"Type":T6, "Method"=→"Method":T7, "output"=→"output":variant)  [unwired: 3 in, 2 out]
      }
      event "update ROI": Value Change {
        n106 = event-data() -> ()  [unwired: 1 in, 6 out]
        n107 = call "myXi_SetParameter.vi"("input PRM"=PRM_v2."WIDTH", "error in"=w274, "input value I32"="Width X", "xiCam IN"=w275) -> ("error out"=w262:errorcluster, "xiCam Out"=w264:refnum<k24>)  [unwired: 6 in]
        n108 = call "myXi_SetParameter.vi"("input PRM"=PRM_v2."HEIGHT", "error in"=w262, "input value I32"="Width Y", "xiCam IN"=w264) -> ("error out"=w261:errorcluster, "xiCam Out"=w263:refnum<k24>)  [unwired: 6 in]
        n109 = call "myXi_SetParameter.vi"("input PRM"=PRM_v2."OFFSET_X", "error in"=w261, "input value I32"="X-offset", "xiCam IN"=w263) -> ("error out"=w269:errorcluster, "xiCam Out"=w267:refnum<k24>)  [unwired: 6 in]
        n110 = call "myXi_SetParameter.vi"("input PRM"=PRM_v2."OFFSET_Y", "error in"=w269, "input value I32"="Y-offset", "xiCam IN"=w267) -> ("error out"=w268:errorcluster)  [unwired: 6 in, 1 out]
      }
      event "data packing": Value Change {
        n111 = event-data() -> ("NewVal"=w281:bool)  [unwired: 1 in, 5 out]
        n112 = case shown="True" w281 {
          tunnel: [i64 0 ("input value I32") i64 1 ("input value I32")] -> w277
          frame False {
          }
          frame True {
          }
        }
        n113 = call "myXi_SetParameter.vi"("input PRM"=PRM_v2."OUTPUT_DATA_PACKING", "error in"=w278, "input value I32"=w277, "xiCam IN"=w280) -> ("error out"=w279:errorcluster)  [unwired: 6 in, 1 out]
      }
      event Value Change {
        n114 = event-data() -> ("NewVal"=w288:T3)  [unwired: 1 in, 5 out]
        n115 = call "IMG_FORMAT - Type.vi"("error in (no error)"=w289, "IMG_FORMAT"=w288) -> ("error out"=w286:errorcluster, "IMG_FORMAT_VALUE"=w287:i32)  [unwired: 8 in]
        n116 = call "myXi_SetParameter.vi"("input PRM"=PRM_v2."IMAGE_DATA_FORMAT", "error in"=w286, "input value I32"=w287, "xiCam IN"=w285) -> ("error out"=w291:errorcluster, "xiCam Out"=w284:refnum<k24>)  [unwired: 6 in]
        n117 = disable-structure shown="Disabled" {
          disable-tunnel: w284 -> [w299 _]
          disable-tunnel: [w298 w300] -> w292
          disable-tunnel: w291 -> [w294 w300]
          disable-tunnel: w288 -> [w293 _]
          frame Disabled {
            n118 = call "IMG_FORMAT - Type.vi"("error in (no error)"=w294, "IMG_FORMAT"=w293) -> ("error out"=w297:errorcluster, "IMG_FORMAT_VALUE"=w296:i32)  [unwired: 8 in]
            n119 = call "myXi_SetParameter.vi"("input PRM"=PRM_v2."IMAGE_DATA_FORMAT_RGB32_ALPHA", "error in"=w297, "input value I32"=w296, "xiCam IN"=w299) -> ("error out"=w298:errorcluster)  [unwired: 6 in, 1 out]
          }
          frame Enabled {
          }
        }
      }
      event "Trigger ON": Value Change {
        n120 = event-data() -> ("NewVal"=w310:bool)  [unwired: 1 in, 5 out]
        n121 = flat-sequence {
          tunnel: w309 -> [w313]
          tunnel: w310 -> [w314]
          tunnel: w311 -> [w315]
          tunnel: [w315] -> w306
          tunnel: [w314] -> w305
          tunnel: [w313] -> w304
          tunnel: [w312] -> w302
          tunnel: [w320] -> w307
          tunnel: w306 -> [w317]
          tunnel: w305 -> [w316]
          tunnel: w304 -> [w321]
          tunnel: [w319] -> w303
          tunnel: w302 -> [w319]
          tunnel: [w318] -> w301
          tunnel: [w322] -> w308
          tunnel: w307 -> [w323]
          tunnel: w303 -> [w325]
          tunnel: w301 -> [w324]
          frame #0 {
            n122 = property on="Play Button" class="Bool (strict)"() -> ("Value"=w312:bool)  [unwired: 2 in, 2 out]
          }
          frame #1 {
            n123 = call "myXi_UpdateTrigger.vi"("error in (no error)"=w321, "trigger"=w316, "xiCam IN"=w317) -> ("error out"=w320:errorcluster, "xiCam Out"=w318:refnum<k24>)  [unwired: 7 in]
          }
          frame #2 {
            n124 = case shown="True" w325 {
              tunnel: w324 -> [_ w329]
              tunnel: w323 -> [w326 w328]
              tunnel: [w326 w327] -> w322
              frame False {
              }
              frame True {
                n125 = invoke class="xiCam" method="StartAcquisition"(reference=w329, error in=w328) -> (error out=w327:errorcluster)  [unwired: 1 in, 2 out]
              }
            }
          }
        }
      }
      event "recent frame": Value Change {
        n126 = event-data() -> ("NewVal"=w333:bool)  [unwired: 1 in, 5 out]
        n127 = case shown="True" w333 {
          tunnel: w332 -> [w335 w343]
          tunnel: w331 -> [w338 w345]
          tunnel: [w337 w344] -> w330
          frame False {
            n128 = call "myXi_SetParameter.vi"("input PRM"=PRM_v2."RECENT_FRAME", "error in"=w338, "input value I32"=0, "xiCam IN"=w335) -> ("error out"=w337:errorcluster)  [unwired: 6 in, 1 out]
          }
          frame True {
            n129 = call "BUFF_POLICY - Type.vi"("BUFF_POLICY"="BUFF_POLICY") -> ("BUFF_POLICY_VALUE"=w339:i32)  [unwired: 9 in, 1 out]
            n130 = call "myXi_SetParameter.vi"("input PRM"=PRM_v2."BUFFER_POLICY", "input value I32"=w339, "xiCam IN"=w343) -> ("xiCam Out"=w341:refnum<k24>)  [unwired: 7 in, 1 out]
            n131 = call "myXi_SetParameter.vi"("input PRM"=PRM_v2."RECENT_FRAME", "error in"=w345, "input value I32"=1, "xiCam IN"=w341) -> ("error out"=w344:errorcluster)  [unwired: 6 in, 1 out]
          }
        }
      }
      event "TIMING MODE": Value Change {
        n132 = event-data() -> ()  [unwired: 1 in, 6 out]
        n133 = call "myXi_SetParameter.vi"("input PRM"=PRM_v2."ACQ_TIMING_MODE", "error in"=w350, "input value I32"="TIMING MODE", "xiCam IN"=w351) -> ("error out"=w349:errorcluster)  [unwired: 6 in, 1 out]
      }
      event "subwindow control": Value Change {
        n134 = event-data() -> ()  [unwired: 1 in, 6 out]
      }
      event "FrameRate": Value Change {
        n135 = event-data() -> ()  [unwired: 1 in, 6 out]
        n136 = call "myXi_SetParameter.vi"("input value DBL"="FrameRate", "input PRM"=PRM_v2."FRAMERATE", "error in"=w356, "xiCam IN"=w357) -> ("error out"=w355:errorcluster)  [unwired: 6 in, 1 out]
      }
      event "software Trigger": Value Change {
        n137 = event-data() -> ()  [unwired: 1 in, 6 out]
        n138 = call "myXi_SetParameter.vi"("input PRM"=PRM_v2."TRG_SOFTWARE", "error in"=w362, "input value I32"=1, "xiCam IN"=w363) -> ("error out"=w359:errorcluster)  [unwired: 6 in, 1 out]
      }
    }
    "command error" <- w204
    n139 = Compound Arithmetic op=ADD(w200, invert w201) -> (w202:dbl)
    n140 = node "Convert Unit"(w202) -> ()  [unwired: 1 out]
  }
  n141 = while {
    tunnel: w22 -> [w379]
    tunnel: [w378] -> w25
    shift-right: [w374] -> _
    shift-left: w26 -> [w371]
    shift-right: [w376] -> _
    shift-left: w21 -> [w366]
    tunnel: w17 -> [w373]
    tunnel: [w372] -> w18
    shift-right: [w368] -> _
    shift-left: w16 -> [w370]
    tunnel: w6 -> [w367]
    stop <- w380 stop-if-true
    # "state machine : slave loop"
    n142 = call <vilib>:"High Resolution Relative Seconds.vi"() -> ("relative seconds"=w365:dbl)
    n143 = case shown="\"acquire sequence\"" w366 {
      tunnel: w379 -> [w388 w393 w399 w428 w500 w568]
      tunnel: [w387 w393 w412 w429 w497 w562] -> w378
      tunnel: [w385 w394 w411 w422 w502 w564] -> w374
      tunnel: [StateMachineControl."wait" ("Enum") StateMachineControl."wait" ("Enum") w403 w433 w496 w569] -> w375
      tunnel: w373 -> [w384 w391 w410 w425 w499 w560]
      tunnel: [w384 w391 w410 w423 w499 w559] -> w372
      tunnel: w371 -> [w386 w394 w402 w432 w503 w567]
      tunnel: w370 -> [w381 w390 w408 w426 w488 w561]
      tunnel: [w381 w390 w409 w431 w491 w558] -> w369
      tunnel: w367 -> [_ _ _ _ w490 _]
      tunnel: w365 -> [_ _ _ w421 _ w556]
      tunnel: [_ _ _ w421 _ w556] -> w364
      frame "stop acquire", Default {
        n144 = call "xiCam - StopAcquisition.vi"("error in (no error)"=w386, "xiCam In"=w388) -> ("error out"=w385:errorcluster, "xiCam Out"=w387:refnum<k24>)  [unwired: 8 in]
        n145 = property on="play sequence" class="Bool (strict)"("Value"=FALSE ("play sequence")) -> ()  [unwired: 2 in, 2 out]
        n146 = property on="Play Button" class="Bool (strict)"("Value"=FALSE ("Play Button")) -> ()  [unwired: 2 in, 2 out]
      }
      frame "wait" {
      }
      frame "start acquire" {
        n147 = control-ref of="Height (def 3424)"() -> (w396:refnum<vi>)
        n148 = call "myXi_GetDataHeight.vi"("Height"=w396, "error in"=w402, "xiCam In"=w399) -> ("error out"=w401:errorcluster, "xiCam Out"=w398:refnum<k24>)  [unwired: 6 in, 1 out]
        n149 = control-ref of="Width (def 4704)"() -> (w395:refnum<vi>)
        n150 = call "myXi_GetDataWidth.vi"("width"=w395, "error in"=w401, "xiCam In"=w398) -> ("error out"=w400:errorcluster, "xiCam Out"=w397:refnum<k24>)  [unwired: 6 in, 1 out]
        n151 = control-ref of="subwindow control"() -> (w405:refnum<vi>)
        n152 = call "myXi_InitializeFreeRunnin.vi"("subimage IN"=w405, "error in (no error)"=w400, "xiCam IN"=w397) -> ("error out"=w404:errorcluster, "Array"=w406:u8[], "xiCam Out"=w407:refnum<k24>)  [unwired: 6 in]
        n153 = case shown="No Error" w404 {
          selector: w404 -> [w414 w420]
          tunnel: [w417 w419] -> w412
          tunnel: [w416 w420] -> w411
          tunnel: w407 -> [w415 w419]
          tunnel: [StateMachineControl."acquire" ("Enum") StateMachineControl."wait" ("Enum")] -> w403
          frame No Error {
            n154 = invoke class="xiCam" method="StartAcquisition"(reference=w415, error in=w414) -> (reference out=w417:refnum<k24>, error out=w416:errorcluster)  [unwired: 1 in, 1 out]
          }
          frame Error {
          }
        }
        n155 = Bundle By Name(cluster=w408, "data array"=w406) -> (w409:T19)
      }
      frame "acquire sequence" {
        n156 = property on="Total sframe" class="DigNum (strict)"() -> ("Value"=w430:i32)  [unwired: 2 in, 2 out]
        n157 = call "myXi_IsSequenceOver.vi"("acquisition frame"=w426, "Max acquisition"=w430, "xiCam In"=w428) -> ("is transfer over ?"=w424:bool, "xiCam Out"=w427:refnum<k24>)  [unwired: 5 in, 2 out]
        n158 = case shown="False" w424 {
          tunnel: [w449 StateMachineControl."stop acquire" ("Enum")] -> w433
          tunnel: w427 -> [w448 w483]
          tunnel: w432 -> [w447 w484]
          tunnel: w426 -> [w444 w482]
          tunnel: [w438 w482] -> w431
          tunnel: [w442 w483] -> w429
          tunnel: w425 -> [w441 w481]
          tunnel: [w440 w481] -> w423
          tunnel: [w437 w484] -> w422
          frame False {
            n159 = call "myXi_AcquireImage.vi"("error in"=w447, "acquisition frame"=w444, "xiCam In"=w448) -> ("error out"=w443:errorcluster, "acquisition frame out"=w439:T19, "xiCam Out"=w442:refnum<k24>, "no Frame Dropped"=w446:bool, "time for acquire"=→"time for acquire":dbl[unit])  [unwired: 4 in]
            n160 = property on="no frame dropping" class="Bool (strict)"("Value"=w446) -> ()  [unwired: 2 in, 2 out]
            n161 = Unbundle By Name(w439) -> ("sframe"=w436:i32)
            "current sequence count" <- w436
            n162 = Greater?(x=w436, y=4) -> (0:w434:bool)
            n163 = case shown="No Error" w443 {
              selector: w443 -> [w453 w466]
              tunnel: [StateMachineControl."acquire sequence" ("Enum") w472] -> w449
              tunnel: [w452 w471] -> w437
              tunnel: w441 -> [w455 w468]
              tunnel: [w454 w468] -> w440
              tunnel: w439 -> [w451 w467]
              tunnel: [w451 w467] -> w438
              tunnel: w434 -> [w450 _]
              frame No Error {
                n164 = case shown="False" w450 {
                  tunnel: w455 -> [w457 w464]
                  tunnel: [w457 w463] -> w454
                  tunnel: w453 -> [w458 w461]
                  tunnel: [w458 w460] -> w452
                  tunnel: w451 -> [_ w459]
                  frame False {
                  }
                  frame True {
                    n165 = Enqueue Element(queue=w464, element=w459, timeout in ms (-1)=1000, error in (no error)=w461) -> (queue out=w463:refnum<queue>, error out=w460:errorcluster)  [unwired: 1 out]
                  }
                }
              }
              frame Error {
                n166 = Unbundle By Name(w467) -> ("sframe"=w470:i32)
                n167 = Unbundle By Name(w466) -> ("code"=w465:i32)
                n168 = Greater Than 0?(x=w470) -> (x > 0?=w469:bool)
                n169 = case shown="0, Default" w465 {
                  tunnel: [StateMachineControl."stop acquire" ("Enum") w478] -> w472
                  tunnel: [w473 errorcluster {"status"=FALSE, "code"=0, "source"=""} ("error IO")] -> w471
                  tunnel: w469 -> [_ w475]
                  tunnel: w466 -> [w473 _]
                  frame 0, Default {
                  }
                  frame 1172 {
                    # "error timeout"
                    n170 = case shown="True" w475 {
                      tunnel: [StateMachineControl."acquire sequence" ("Enum") StateMachineControl."stop acquire" ("Enum")] -> w478
                      frame False {
                      }
                      frame True {
                      }
                    }
                    "timeout" <- TRUE
                  }
                }
              }
            }
          }
          frame True {
          }
        }
      }
      frame "start acquire sequence" {
        w489 = 0 ("sframe")
        n171 = control-ref of="Height (def 3424)"() -> (w498:refnum<vi>)
        n172 = control-ref of="Width (def 4704)"() -> (w501:refnum<vi>)
        n173 = control-ref of="subwindow control"() -> (w486:refnum<vi>)
        n174 = call "myXi_GetDataHeight.vi"("Height"=w498, "error in"=w503, "xiCam In"=w500) -> ("error out"=w504:errorcluster, "xiCam Out"=w505:refnum<k24>)  [unwired: 6 in, 1 out]
        n175 = call "myXi_GetDataWidth.vi"("width"=w501, "error in"=w504, "xiCam In"=w505) -> ("error out"=w494:errorcluster, "xiCam Out"=w495:refnum<k24>)  [unwired: 6 in, 1 out]
        n176 = disable-structure shown="Enabled" {
          disable-tunnel: w495 -> [w512 w518]
          disable-tunnel: w494 -> [w511 w515]
          disable-tunnel: [w510 w517] -> w493
          disable-tunnel: [w509 w513] -> w492
          disable-tunnel: [w507 w516] -> w487
          disable-tunnel: w486 -> [w506 w514]
          frame Enabled {
            n177 = call "myXi_InitializeStartBust.vi"("subwindow IN"=w506, "error in (no error)"=w511, "image frames"="buffer frames", "xiCam IN"=w512) -> ("error out"=w507:errorcluster, "Array"=w509:u8[], "xiCam Out"=w510:refnum<k24>)  [unwired: 5 in]
          }
          frame Disabled {
            n178 = call "myXi_InitializeFreeRunnin.vi"("subimage IN"=w514, "error in (no error)"=w515, "xiCam IN"=w518) -> ("error out"=w516:errorcluster, "Array"=w513:u8[], "xiCam Out"=w517:refnum<k24>)  [unwired: 6 in]
          }
        }
        n179 = Bundle By Name(cluster=w488, "sframe"=w489, "data array"=w492) -> (w491:T19)
        n180 = case shown="No Error" w487 {
          selector: w487 -> [w519 w554]
          tunnel: [w525 w554] -> w502
          tunnel: [w524 w555] -> w497
          tunnel: [w523 StateMachineControl."wait" ("Enum")] -> w496
          tunnel: w493 -> [w522 w555]
          tunnel: w490 -> [w521 _]
          tunnel: w489 -> [w520 _]
          frame No Error {
            n181 = flat-sequence {
              tunnel: w519 -> [w533]
              tunnel: w522 -> [w534]
              tunnel: [w534] -> w529
              tunnel: [w533] -> w528
              tunnel: w521 -> [w532]
              tunnel: w520 -> [_]
              tunnel: [w535] -> w527
              tunnel: [w537] -> w526
              tunnel: w529 -> [w538]
              tunnel: w528 -> [w536]
              tunnel: [w540] -> w524
              tunnel: [w541] -> w525
              tunnel: w527 -> [w539]
              tunnel: w526 -> [w542]
              tunnel: [StateMachineControl."acquire sequence" ("Enum")] -> w523
              frame #0 {
                n182 = Wait on Occurrence(1:FALSE ("ignore previous (T)"), 2:w532, 3:5000 ("ms timeout (-1)")) -> ()  [unwired: 1 out]
              }
              frame #1 {
                n183 = invoke class="xiCam" method="StartAcquisition"(reference=w538, error in=w536) -> (reference out=w537:refnum<k24>, error out=w535:errorcluster)  [unwired: 1 in, 1 out]
              }
              frame #2 {
                n184 = disable-structure shown="Enabled" {
                  disable-tunnel: w542 -> [w548 w552]
                  disable-tunnel: [w547 w551] -> w541
                  disable-tunnel: [w546 w552] -> w540
                  disable-tunnel: w539 -> [w545 w551]
                  frame Disabled {
                    n185 = call "myXi_SetParameter.vi"("input PRM"=PRM_v2."TRG_SOFTWARE", "error in"=w545, "input value I32"=1, "xiCam IN"=w548) -> ("error out"=w547:errorcluster, "xiCam Out"=w546:refnum<k24>)  [unwired: 6 in]
                  }
                  frame Enabled {
                  }
                }
                n186 = Wait (ms)(milliseconds to wait=u32 200) -> ()  [unwired: 1 out]
              }
            }
          }
          frame Error {
          }
        }
      }
      frame "acquire" {
        n187 = call "myXi_AcquireImage.vi"("error in"=w567, "acquisition frame"=w561, "xiCam In"=w568) -> ("error out"=w566:errorcluster, "acquisition frame out"=w558:T19, "xiCam Out"=w563:refnum<k24>, "no Frame Dropped"=→"no frame dropping":bool, "time for acquire"=→"time for acquire":dbl[unit])  [unwired: 4 in]
        n188 = invoke class="xiCam" method="GetLastImageParams"(reference=w563) -> (reference out=w562:refnum<k24>)  [unwired: 2 in, 2 out]
        n189 = case shown="No Error" w566 {
          selector: w566 -> [w575 w579]
          tunnel: [StateMachineControl."acquire" ("Enum") w581] -> w569
          tunnel: [w575 w578] -> w564
          tunnel: w560 -> [w574 w577]
          tunnel: [w573 w577] -> w559
          tunnel: w558 -> [w572 _]
          frame No Error {
            n190 = Bundle By Name(cluster=w572, "is sequence running ?"=FALSE) -> (w570:T19)
            n191 = Enqueue Element(queue=w574, element=w570) -> (queue out=w573:refnum<queue>)  [unwired: 2 in, 2 out]
          }
          frame Error {
            n192 = Unbundle By Name(w579) -> ("code"=w580:i32)
            n193 = case shown="1172" w580 {
              tunnel: [StateMachineControl."wait" ("Enum") StateMachineControl."acquire" ("Enum")] -> w581
              tunnel: [w582 errorcluster {"status"=FALSE, "code"=0, "source"=""} ("error IO")] -> w578
              tunnel: w579 -> [w582 _]
              frame 0, Default {
              }
              frame 1172 {
              }
            }
          }
        }
      }
    }
    "error out" <- w374
    n194 = event shown="[1] \"Play Button\": Value Change" {
      selector: _ -> [_ _ _ _ _ _]
      dyn-events: _ -> [_ _ _ _ _ _]
      timeout: 0 -> [_ _ _ _ _ _]
      tunnel: [_ _ _ _ TRUE _] -> w380
      tunnel: [w591 w593 w598 StateMachineControl."stop acquire" ("Enum") StateMachineControl."wait" ("Enum") w607] -> w376
      tunnel: w375 -> [w591 _ _ _ _ w607]
      tunnel: w369 -> [w590 w592 w597 w602 w604 w608]
      tunnel: [w590 w592 w597 w602 w604 w608] -> w368
      tunnel: w364 -> [w586 _ _ _ _ _]
      event Timeout {
        n195 = event-data() -> ()  [unwired: 1 in, 3 out]
        n196 = call <vilib>:"High Resolution Relative Seconds.vi"() -> ("relative seconds"=w587:dbl)
        n197 = Compound Arithmetic op=ADD(w587, invert w586) -> (w589:dbl)
        n198 = node "Convert Unit"(w589) -> (→"loop":dbl[unit])
      }
      event "Play Button": Value Change {
        n199 = event-data() -> ("NewVal"=w594:bool)  [unwired: 1 in, 3 out]
        n200 = case shown="True" w594 {
          tunnel: [StateMachineControl."stop acquire" ("Enum") StateMachineControl."start acquire" ("Enum")] -> w593
          frame False {
          }
          frame True {
          }
        }
      }
      event "play sequence": Value Change {
        n201 = event-data() -> ("NewVal"=w599:bool)  [unwired: 1 in, 5 out]
        n202 = case shown="True" w599 {
          tunnel: [StateMachineControl."stop acquire" ("Enum") StateMachineControl."start acquire sequence" ("Enum")] -> w598
          frame False {
          }
          frame True {
          }
        }
      }
      event "update loop": Value Change {
        n203 = event-data() -> ()  [unwired: 1 in, 6 out]
      }
      event "Stop Button": Value Change {
        n204 = event-data() -> ()  [unwired: 1 in, 5 out]
      }
      event "Trigger ON": Value Change {
        (unwired) StateMachineControl."stop acquire" ("Enum")
        n205 = event-data() -> ()  [unwired: 1 in, 6 out]
      }
    }
    "Enum" <- w366
  }
  n206 = disable-structure shown="Disabled" {
    disable-tunnel: [w610 _] -> w10
    disable-tunnel: [w609 _] -> w9
    frame Disabled {
      n207 = flat-sequence {
        tunnel: [w611] -> _
        tunnel: [w613] -> w609
        tunnel: [w611] -> w610
        frame #0 {
          # "open network shared variables"
          n208 = shared-variable-open(refnum<k21> "ni.var.psp://localhost/MySharedVariables/MasterStatusShared" ("shared variable refnum in"), T25 [] ("Master Status")) -> (w611:refnum<k21>, w613:errorcluster)  [unwired: 2 in]
        }
      }
    }
    frame Enabled {
    }
  }
  n209 = while {
    tunnel: w17 -> [w639]
    tunnel: [w639] -> _
    tunnel: [w636] -> w12
    tunnel: [w635] -> w11
    tunnel: w10 -> [w634]
    tunnel: w9 -> [w633]
    tunnel: w8 -> [w626]
    tunnel: w7 -> [w627]
    tunnel: w6 -> [w629]
    shift-right: [w624] -> _
    shift-left: w4 -> [w623]
    shift-right: [w616] -> _
    shift-left: w5 -> [w630]
    shift-right: [w621] -> _
    shift-left: _ -> [w620]
    stop <- w628 stop-if-true
    # "data analysis slave loop"
    n210 = event shown="[11] \"Save As Button\": Value Change" {
      selector: _ -> [_ _ _ _ _ _ _ _ _ _ _ _ _ _ _ _ _]
      dyn-events: _ -> [_ _ _ _ _ _ _ _ _ _ _ _ _ _ _ _ _]
      timeout: 0 -> [_ _ _ _ _ _ _ _ _ _ _ _ _ _ _ _ _]
      tunnel: w639 -> [w683 w694 w698 w709 w712 w722 w729 w736 w745 w749 w762 w766 w770 w774 w776 w782 w786]
      tunnel: [w682 w694 w698 w709 w712 w722 w729 w736 w745 w749 w762 w766 w770 w774 w776 w782 w786] -> w638
      tunnel: [w680 w691 w696 w708 _ w717 w723 w733 w744 w746 w750 w763 w767 w771 w775 w779 w783] -> w637
      tunnel: w630 -> [w673 _ _ _ w710 w718 _ w735 w742 _ w751 w764 _ _ _ _ _]
      tunnel: w629 -> [_ _ w702 _ _ _ _ _ _ _ _ _ _ _ _ _ _]
      tunnel: [_ TRUE _ _ _ _ _ _ _ _ _ _ _ _ _ _ _] -> w628
      tunnel: w627 -> [_ _ _ _ _ _ _ _ _ _ _ _ _ _ _ _ _]
      tunnel: w626 -> [_ _ _ _ _ _ _ _ _ _ _ _ _ _ _ _ _]
      tunnel: [w674 w693 w700 w706 w711 w719 w727 _ w743 w748 _ _ w769 w773 w777 w781 w785] -> w625
      tunnel: w623 -> [w674 w693 w700 w706 w711 w719 _ _ w743 w748 _ _ _ w773 w777 w781 w785]
      tunnel: [w673 StateProcessingLoop."free run" ("Enum") w699 StateProcessingLoop."free run" ("NewVal") w710 w718 w728 w735 w742 StateProcessingLoop."network sequence" ("Enum") w751 w764 w768 StateProcessingLoop."Snap BG" ("NewVal") StateProcessingLoop."Snap REF" ("NewVal") StateProcessingLoop."Snap MAIN" ("NewVal") StateProcessingLoop."Snap REF+MAIN" ("NewVal")] -> w622
      tunnel: w620 -> [_ w691 w696 w708 _ w717 w723 w733 w744 w746 w750 w763 w767 w771 w775 w779 w783]
      event Timeout {
        n211 = event-data() -> ()  [unwired: 1 in, 3 out]
        n212 = property on="unit" class="Enum (strict)"() -> ("Value"=w671:T14)  [unwired: 2 in, 2 out]
        n213 = Get Queue Status(queue=w683) -> (queue out=w682:refnum<queue>, error out=w681:errorcluster, # elements in queue=w679:i32)  [unwired: 2 in, 5 out]
        "# elements queue" <- w679
        n214 = case shown="\"Efficiency\"" w671 {
          tunnel: ["average Nphotons" ("Label.Text") "average Efficiency" ("Label.Text") "uW" ("Label.Text") "nW" ("Label.Text") "Nelectrons" ("Label.Text") "W" ("Label.Text") "average Ncounts" ("Label.Text")] -> w672
          frame "Nphotons" {
          }
          frame "Efficiency" {
          }
          frame "I(uW/cm^2)" {
          }
          frame "I(nW/cm^2)" {
          }
          frame "Nelectrons" {
          }
          frame "I[W/cm^2]" {
          }
          frame "counts", Default {
          }
        }
        "unit" <- w672
        n215 = Greater Than 0?(x=w679) -> (x > 0?=w678:bool)
        n216 = Select(t=errorcluster {"status"=FALSE, "code"=0, "source"=""} ("error constant"), s=w678, f=errorcluster {"status"=TRUE, "code"=0, "source"=""} ("error constant")) -> (s? t:f=w675:errorcluster)
        n217 = Merge Errors(w681, w675) -> (w680:errorcluster)
      }
      event "Stop Button": Value Change {
        n218 = event-data() -> ()  [unwired: 1 in, 6 out]
      }
      event "play sequence": Value Change {
        n219 = event-data() -> ()  [unwired: 1 in, 6 out]
        n220 = flat-sequence {
          tunnel: w702 -> [w704]
          tunnel: [w704] -> w701
          tunnel: [StateProcessingLoop."sequence" ("Enum")] -> w699
          tunnel: w701 -> [w705]
          frame #0 {
          }
          frame #1 {
            n221 = Set Occurrence(w705) -> ()
          }
        }
        n222 = local write "Array"(i32[] [] ("Array")) -> ()
      }
      event "Play Button": Value Change {
        n223 = event-data() -> ()  [unwired: 1 in, 6 out]
      }
      event "Save result": Value Change {
        n224 = event-data() -> ()  [unwired: 1 in, 6 out]
        n225 = property on="result array" class="Arr (strict)"() -> ("Value"=w714:dbl[][])  [unwired: 2 in, 2 out]
        n226 = call "SaveArray.vi"("name or relative path"="name 2", "saving folder"="Target Folder 2", "overwrite"=TRUE, "array"=w714) -> ()  [unwired: 7 in, 1 out]
      }
      event "clear graph": Value Change {
        n227 = event-data() -> ()  [unwired: 1 in, 6 out]
        n228 = control-ref of="Waveform Chart"() -> (w721:refnum<vi>)
        n229 = property class="WFChart (strict)"(reference=w721, "History Data"=waveform(dbl)[] []) -> ()  [unwired: 1 in, 2 out]
      }
      event "start stats": Value Change {
        n230 = event-data() -> ()  [unwired: 1 in, 6 out]
        n231 = case shown="True" "start stats" {
          tunnel: [StateProcessingLoop."free run" ("Enum") StateProcessingLoop."statistics" ("Enum")] -> w728
          frame False {
          }
          frame True {
          }
        }
        n232 = property on="subwindow control" class="Clust (strict)"() -> ("Value"=w724:T10)  [unwired: 2 in, 2 out]
        n233 = call "WindowsClusterToSize.vi"("subwindow control 2"=w724) -> ("Ny"=w725:dbl, "Nx"=w726:dbl)  [unwired: 9 in]
        n234 = call "InitAnalysesVariables.vi"("Ny [rows]"=w725, "Nx [cols]"=w726) -> ("Stat Vars"=w727:T23)  [unwired: 9 in]
      }
      event "default BG": Value Change {
        n235 = event-data() -> ()  [unwired: 1 in, 6 out]
        n236 = property on="subwindow control" class="Clust (strict)"() -> ("Value"=w734:T10)  [unwired: 2 in, 2 out]
        n237 = call "SetGlobalToZero.vi"("subwindow control"=w734) -> ()  [unwired: 11 in]
      }
      event "view snaps": Value Change {
        n238 = event-data() -> ()  [unwired: 1 in, 6 out]
        n239 = global read "References.vi" "Ref only"() -> (w739:dbl[][])
        n240 = global read "References.vi" "Background"() -> (w740:dbl[][])
        n241 = global read "References.vi" "Main only"() -> (w741:dbl[][])
        n242 = Subtract(x=w739, y=w740) -> (x-y=w738:dbl[][])
        n243 = Subtract(x=w741, y=w740) -> (x-y=w737:dbl[][])
        n244 = property on="MAIN" class="IntGraph (strict)"("Value"=w737) -> ()  [unwired: 2 in, 2 out]
        n245 = property on="BG" class="IntGraph (strict)"("Value"=w740) -> ()  [unwired: 2 in, 2 out]
        n246 = property on="REF" class="IntGraph (strict)"("Value"=w738) -> ()  [unwired: 2 in, 2 out]
      }
      event "start network scan": Value Change {
        n247 = event-data() -> ()  [unwired: 1 in, 6 out]
      }
      event "subwindow control": Value Change {
        w753 = 0.005 ("input X")
        n248 = event-data() -> ("NewVal"=w752:T10)  [unwired: 1 in, 5 out]
        n249 = control-ref of="Intensity Graph"() -> (w761:refnum<vi>)
        n250 = call "UpdateFFTwindow.vi"("subwindow IN"=w752, "Intensity Graph"=w761) -> ("output cluster"=w756:T9)  [unwired: 9 in]
        n251 = Unbundle By Name(w756) -> ("X"=w757:dbl, "Y"=w758:dbl)
        n252 = call "BuilFFT_cluster.vi"("Enum"=enum16{"by dF", "by dX"}."by dX", "input Y"=w753, "input X"=w753, "Ny"=w758, "Nx"=w757) -> ("fft cluster"=w760:T16)  [unwired: 6 in]
        n253 = property on="fft cluster" class="Clust (strict)"("Value"=w760) -> ()  [unwired: 2 in, 2 out]
        n254 = control-ref of="FFT"() -> (w759:refnum<vi>)
        n255 = call "RescaleGraphForFourier.vi"("fft reference"=w759, "fft cluster"=w760, "Enum"=enum16{"Reciprocal", "Real"}."Reciprocal") -> ()  [unwired: 8 in]
      }
      event "Save As Button": Value Change {
        n256 = event-data() -> ()  [unwired: 1 in, 6 out]
        n257 = property on="Intensity Graph" class="IntGraph (strict)"() -> ("Value"=w765:u16[][])  [unwired: 2 in, 2 out]
        n258 = call "SaveAsArrayTiff.vi"("u16 array"=w765) -> ()  [unwired: 11 in]
      }
      event Value Change {
        n259 = event-data() -> ("NewVal"=w768:T2)  [unwired: 1 in, 5 out]
        n260 = call "InitAnalysesVariables.vi"() -> ("Stat Vars"=w769:T23)  [unwired: 11 in]
      }
      event "Snap": Value Change {
        n261 = event-data() -> ()  [unwired: 1 in, 6 out]
      }
      event "Snap 2": Value Change {
        n262 = event-data() -> ()  [unwired: 1 in, 6 out]
      }
      event "Snap 3": Value Change {
        n263 = event-data() -> ()  [unwired: 1 in, 6 out]
      }
      event "Snap 4": Value Change {
        n264 = event-data() -> ()  [unwired: 1 in, 6 out]
      }
    }
    n265 = property on="subwindow control" class="Clust (strict)"() -> ("Value"=w632:T10)  [unwired: 2 in, 2 out]
    n266 = case shown="No Error" w637 {
      selector: w637 -> [_ w966]
      tunnel: w638 -> [w812 _]
      tunnel: [w807 w969] -> w636
      tunnel: [w806 w968] -> w635
      tunnel: w634 -> [w805 w969]
      tunnel: w633 -> [w804 w968]
      tunnel: w632 -> [w803 _]
      tunnel: w625 -> [w801 w967]
      tunnel: [w802 w967] -> w624
      tunnel: w622 -> [w798 w965]
      tunnel: [w800 w965] -> w616
      tunnel: [_ w966] -> w621
      tunnel: ["auto-save ?" FALSE ("auto-save ?")] -> w619
      tunnel: [w795 0 ("nframe")] -> w618
      tunnel: [w794 u16[][] [] ("output array")] -> w617
      tunnel: [w792 w961] -> w615
      frame No Error {
        n267 = property on="Width (def 4704)" class="DigNum (strict)"() -> ("Value"=w809:i32)  [unwired: 2 in, 2 out]
        n268 = property on="Height (def 3424)" class="DigNum (strict)"() -> ("Value"=w810:i32)  [unwired: 2 in, 2 out]
        n269 = Dequeue Element(queue=w812, timeout in ms (-1)=1000) -> (element=w808:T19)  [unwired: 1 in, 3 out]
        n270 = call "myXi_ReshapeArray.vi"("width"=w809, "height"=w810, "acquisition frame"=w808) -> ("output array"=w794:u16[][])  [unwired: 8 in]
        "Intensity Graph" <- w794
        n271 = Unbundle By Name(w808) -> ("nframe"=w791:i32, "timestamp"=w793:dbl)
        "timestamp" <- w793
        n272 = case shown="True" "data analysis on" {
          tunnel: w793 -> [_ w832]
          tunnel: w794 -> [_ w831]
          tunnel: w803 -> [_ w830]
          tunnel: w798 -> [_ w827]
          tunnel: [StateProcessingLoop."free run" ("NewVal") w827] -> w797
          tunnel: [0.0 ("Ptot") w820] -> w790
          tunnel: [0.0 ("variance coeff") w819] -> w789
          tunnel: [_ w816] -> w788
          tunnel: [_ w817] -> w787
          frame False {
          }
          frame True {
            n273 = control-ref of="FFT"() -> (w829:refnum<vi>)
            n274 = property on="fft cluster" class="Clust (strict)"() -> ("Value"=w828:T16)  [unwired: 2 in, 2 out]
            n275 = call "reshapeAndExtract.vi"("window"=w830, "output array"=w831) -> ("subarray"=w817:dbl[][])  [unwired: 9 in]
            n276 = control-ref of="Ptot"() -> ()  [unwired: 1 out]
            n277 = Bundle("Filter on/off"="Filter on/off", "filtered int/phase"="filtered int/phase", "Mask ON"="Mask ON", "FFT int/phase"="FFT int/phase") -> (w833:T27)  [unwired: 1 in]
            n278 = case shown="True" "minus BG" {
              tunnel: [w845 w846] -> w821
              tunnel: w817 -> [w845 w847]
              frame False {
              }
              frame True {
                n279 = global read "References.vi" "Background"() -> (w848:dbl[][])
                n280 = Subtract(x=w847, y=w848) -> (x-y=w846:dbl[][])
              }
            }
            n281 = call "GetTaggedPhotons.vi"("screen status"=w833, "fft cluster"=w828, "FFT reference"=w829, "unit"="unit", "I (current unit)"=w821) -> ("output cluster 2"=w825:T28)  [unwired: 6 in]
            n282 = Unbundle By Name(w825) -> ("Ifft"=→"FFT":dbl[][], "Tagged Photons"=w816:dbl[][], "% saturation"=→"% saturation":dbl, "Ptot"=w820:dbl, "efficiency"=→"efficiency to Main":dbl, "variance coeff"=w819:dbl)
            "Ptot" <- w820
            "filtered  FFT" <- w816
            n283 = disable-structure shown="Enabled" {
              disable-tunnel: w832 -> [w840 _]
              disable-tunnel: w820 -> [w838 w843]
              frame Disabled {
                n284 = control-ref of="Waveform Chart"() -> (w839:refnum<vi>)
                n285 = call "DataWaveformChart.vi"("FFT full energy"=w838, "timestamp"=w840, "waveform chart"=w839) -> ()  [unwired: 9 in]
              }
              frame Enabled {
                n286 = Not(x="Pause log") -> (.not. x?=w841:bool)
                n287 = case shown="True" w841 {
                  tunnel: w843 -> [_ w844]
                  frame False {
                  }
                  frame True {
                    "Waveform Chart" <- w844
                  }
                }
              }
            }
          }
        }
        n288 = case shown="\"statistics\"" w797 {
          selector: w797 -> [w854 w863 w884 _ _ _ _ _]
          tunnel: w808 -> [w858 _ _ _ _ _ _ _]
          tunnel: [w857 w866 w886 w913 w940 w946 w952 w958] -> w807
          tunnel: [w856 w865 w885 w912 w941 w945 w953 w957] -> w806
          tunnel: w805 -> [w857 w866 w886 w911 w940 w946 w952 w958]
          tunnel: w804 -> [w856 w865 w885 w910 w941 w945 w953 w957]
          tunnel: w801 -> [w855 w864 w880 w909 w942 w947 w951 w959]
          tunnel: [w855 w864 w879 w909 w942 w947 w951 w959] -> w802
          tunnel: [w854 w863 w874 w907 StateProcessingLoop."free run" ("Enum") StateProcessingLoop."free run" ("Enum") StateProcessingLoop."free run" ("Enum") StateProcessingLoop."free run" ("Enum")] -> w800
          tunnel: w791 -> [w853 w862 w873 w906 w938 w944 w950 w956]
          tunnel: [w853 w862 w873 w906 w938 w944 w950 w956] -> w795
          tunnel: [w849 _ _ _ _ _ _ _] -> w792
          tunnel: w790 -> [_ _ w872 _ _ _ _ _]
          tunnel: w789 -> [_ _ w870 _ _ _ _ _]
          tunnel: w788 -> [_ _ w867 _ _ _ _ _]
          tunnel: w787 -> [_ _ _ _ w937 w943 w949 w955]
          frame "sequence", Default {
            n289 = property on="sequence cluster" class="Clust (strict)"() -> ("Value"=w860:T17)  [unwired: 2 in, 2 out]
            n290 = Unbundle By Name(w860) -> ("Nevent"=w859:i32)
            n291 = call "GetFrameFFT_index.vi"("sframe Max"=w859, "element"=w858) -> ("index out"=w850:i32)  [unwired: 8 in, 1 out]
            n292 = local read "Array"() -> (w852:i32[])
            n293 = call "unwrapSequence.vi"("result array in"="result array", "index in"=w850) -> ("result array out"=w849:dbl[][])  [unwired: 9 in]
            n294 = Insert Into Array(array=w852, new element=w850) -> (w851:i32[])  [unwired: 1 in]
            n295 = local write "Array"(w851) -> ()
            n296 = property on="result array" class="Arr (strict)"("Value"=w849) -> ()  [unwired: 2 in, 2 out]
          }
          frame "free run" {
          }
          frame "statistics" {
            n297 = case shown="True" FALSE {
              tunnel: w884 -> [w891 _]
              tunnel: [w891 StateProcessingLoop."free run" ("Enum")] -> _
              frame False {
              }
              frame True {
                # "save stats"
                n298 = call "FetchTargetFolder.vi"() -> ("error out"=w897:errorcluster, "Full File Path"=w896:path)  [unwired: 10 in]
                n299 = Concatenate Strings("save name", "_mu" ("string")) -> (w903:string)
                n300 = Concatenate Strings("save name", "_std" ("string")) -> (w898:string)
                n301 = call "FetchTargetFile.vi"("file type"=FileType."tiff", "error in (no error)"=w897, "FileName"=w903, "Target Folder"=w896) -> ("error out"=w892:errorcluster, "Full File Path"=w895:path)  [unwired: 6 in]
                n302 = call "FetchTargetFile.vi"("file type"=FileType."tiff", "error in (no error)"=w897, "FileName"=w898, "Target Folder"=w896) -> ("error out"=w893:errorcluster, "Full File Path"=w894:path)  [unwired: 6 in]
                n303 = call "SaveArrayTiff.vi"("Target Folder"=w895, "error in (no error)"=w892) -> ()  [unwired: 9 in, 1 out]
                n304 = call "SaveArrayTiff.vi"("Target Folder"=w894, "error in (no error)"=w893) -> ()  [unwired: 9 in, 1 out]
              }
            }
            n305 = call "StatisticsFromArray.vi"("Naverage"="Naverage 2D", "input Ptot"=w872, "input VAR"=w867, "Stat Vars"=w880) -> ("STD"=→"STD":dbl[][], "MU"=→"MU":dbl[][], "VAR(n+1)"=w879:T23, "std"=→"std":dbl, "mu"=w871:dbl)  [unwired: 3 in]
            "mu" <- w871
            n306 = Multiply(x=w870, y=w871) -> (x*y=w869:dbl)
            n307 = Square Root(x=w869) -> (sqrt(x)=→"shot noise std":dbl)
            n308 = Unbundle By Name(w879) -> ("n"=w877:i32)
            "n" <- w877
            n309 = Greater?(x=w877, y="Naverage 2D") -> (0:w875:bool)
            n310 = case shown="True" w875 {
              tunnel: [StateProcessingLoop."statistics" ("Enum") StateProcessingLoop."free run" ("Enum")] -> w874
              frame False {
              }
              frame True {
                n311 = control-ref of="start stats"() -> (w888:refnum<vi>)
                n312 = property class="Bool (strict)"(reference=w888, "Value"=FALSE) -> ()  [unwired: 1 in, 2 out]
              }
            }
          }
          frame "network sequence" {
            n313 = case shown="True" FALSE {
              tunnel: [StateProcessingLoop."network sequence" ("Enum") StateProcessingLoop."free run" ("Enum")] -> w907
              tunnel: [w915 w921] -> w913
              tunnel: [w914 w920] -> w912
              tunnel: w911 -> [w915 w919]
              tunnel: w910 -> [w914 w918]
              frame False {
              }
              frame True {
                n314 = flat-sequence {
                  tunnel: [w923] -> w917
                  tunnel: [w923] -> _
                  tunnel: [w929] -> w921
                  tunnel: [w928] -> w920
                  tunnel: w919 -> [w927]
                  tunnel: w918 -> [w926]
                  tunnel: w917 -> [w925]
                  frame #0 {
                    # "edit labview chart"
                    n315 = property on="Sequence Number" class="DigNum (strict)"() -> ("Value"=w923:u64)  [unwired: 2 in, 2 out]
                  }
                  frame #1 {
                    # "indicate ready"
                    n316 = property on="start network scan" class="Bool (strict)"("Value"=FALSE ("start network scan")) -> ()  [unwired: 2 in, 2 out]
                    n317 = shared-variable-read(w927, w926) -> (w932:refnum<k21>, w931:errorcluster, w930:T25)  [unwired: 1 out]
                    n318 = in-place {
                      n319 = in-place-array #1(w930, w925) -> (w936:T29)
                      n320 = Bundle By Name(cluster=w936, "Camera done"=TRUE) -> (w934:T29)
                      n321 = in-place-array #1(w934) -> (w924:T25)  [unwired: 1 out]
                    }
                    n322 = shared-variable-write(w932, w931, w924) -> (w929:refnum<k21>, w928:errorcluster)
                  }
                }
              }
            }
          }
          frame "Snap REF+MAIN" {
            "REF+MAIN" <- w937
          }
          frame "Snap MAIN" {
            n323 = global write "References.vi" "Main only"(w943) -> ()
            "MAIN" <- w943
          }
          frame "Snap REF" {
            n324 = global write "References.vi" "Ref only"(w949) -> ()
            "REF" <- w949
          }
          frame "Snap BG" {
            n325 = global write "References.vi" "Background"(w955) -> ()
            "BG" <- w955
          }
        }
      }
      frame Error {
        n326 = property on="result array" class="Arr (strict)"() -> ("Value"=w961:dbl[][])  [unwired: 2 in, 2 out]
      }
    }
    n327 = case shown="\"sequence\", Default" w616 {
      tunnel: w615 -> [w645 _ _ _ _ _ _ _]
      frame "sequence", Default {
        n328 = property on="sequence cluster" class="Clust (strict)"() -> ("Value"=w644:T17)  [unwired: 2 in, 2 out]
        n329 = Unbundle By Name(w644) -> ("TypeOfSequence"=w643:string)
        n330 = case shown="\"JM\", Default" w643 {
          tunnel: w645 -> [w649 w658]
          tunnel: "fft cluster acquisition" -> [w648 w652]
          tunnel: [w647 w651] -> w641
          tunnel: [w646 w650] -> w640
          frame "OFJM" {
            n331 = call "ZFFTunwrappedResult.vi"("fft cluster acquisition"=w648, "result array out"=w649) -> ("image"=w646:dbl[][], "modules FFT"=w647:dbl[][])  [unwired: 8 in]
          }
          frame "JM", Default {
            w659 = 1000.0 ("x")
            n332 = Bundle("phi(1) X"="phi(1) X", "phi(1) Z"="phi(1) Z", "phi(2) X"="phi(2) X", "phi(2) Z"="phi(2) Z") -> (w653:T30)  [unwired: 1 in]
            n333 = call "FFTunwrappedResult.vi"("fft cluster acquisition"=w652, "sequence NbX NbZ"="sequence NbX NbZ", "output cluster"=w653, "result array out"=w658) -> ("image"=w650:dbl[][], "modules FFT"=w651:dbl[][])  [unwired: 6 in]
            n334 = Unbundle By Name(w652) -> ("dx"=w661:dbl, "dy"=w664:dbl)
            n335 = Multiply(x=w659, y=w661) -> (x*y=w662:dbl)
            n336 = Multiply(x=w659, y=w664) -> (x*y=w663:dbl)
            n337 = property on="reconstructed image" class="IntGraph (strict)"("XScale.Multiplier"=w662, "YScale.Multiplier"=w663) -> ()  [unwired: 2 in, 2 out]
          }
        }
        "FFT acquire Graph" <- w641
        "reconstructed image" <- w640
      }
      frame "Snap REF+MAIN" {
      }
      frame "Snap MAIN" {
      }
      frame "Snap REF" {
      }
      frame "Snap BG" {
      }
      frame "network sequence" {
      }
      frame "free run" {
      }
      frame "statistics" {
      }
    }
    n338 = case shown="True" w619 {
      tunnel: w626 -> [_ w668]
      tunnel: w618 -> [_ w667]
      tunnel: w617 -> [_ w666]
      frame False {
      }
      frame True {
        n339 = call "SaveArrayTiff.vi"("name"="name", "Target Folder"=w668, "output array"=w666, "number"=w667) -> ("error out"=w665:errorcluster)  [unwired: 7 in]
        n340 = case shown="Error" w665 {
          frame No Error {
          }
          frame Error {
            n341 = property on="auto-save ?" class="Bool (strict)"("Value"=FALSE ("auto-save ?")) -> ()  [unwired: 2 in, 2 out]
          }
        }
      }
    }
    "status analysis" <- w630
  }
  n342 = flat-sequence {
    tunnel: w25 -> [w973]
    tunnel: w18 -> [w972]
    frame #0 {
      w971 = FALSE ("Play Button")
      # "exit"
      n343 = call "xiCam - CloseDevice.vi"("xiCam In"=w973) -> ()  [unwired: 10 in, 1 out]
      n344 = Release Queue(queue=w972) -> ()  [unwired: 2 in, 3 out]
      n345 = property on="Play Button" class="Bool (strict)"("Value"=w971) -> ()  [unwired: 2 in, 2 out]
      n346 = property on="play sequence" class="Bool (strict)"("Value"=w971) -> ()  [unwired: 2 in, 2 out]
      n347 = property on="start stats" class="Bool (strict)"("Value"=FALSE ("start stats")) -> ()  [unwired: 2 in, 2 out]
    }
  }
  n348 = Close Variable Connection(8:w11, 11:w12) -> ()  [unwired: 1 out]
